vi "AutoBurn-BMU.vi"(0 "类型":u32(ring)=4 items=["PCI5121"=1, "PCI9810"=2, "USBCAN1"=3, "USBCAN2"=4, "PCI9820"=5, "CAN232"=6, "PCI5110"=7, "CANLite(mini)"=8, "ISA9620"=9, "ISA5420"=10, "PC104CAN"=11, "CANET"=17, "DNP9810"=13, "USBCAN-E-U"=20, "USBCAN-2E-U"=21], 1 "MyIndex":i32, 5 "波特率":T2(ring)=enum."500Kbps", 7 "设备索引":u32(ring) items=["0", "1", "2", "3", "4", "5", "6", "7", "8", "9", "10", "11", "12", "13", "14", "15", ""], 9 "CAN路数":u32(ring) items=["0", "1"], 11 "请选择板号":u16(ring)=1 items=["BMU1"=1, "BMU2"=2, "BMU3"=3, "BMU4"=4, "BMU5"=5, "BMU6"=6, "BMU7"=7, "BMU8"=8, "BMU9"=9, "BMU10"=10, "BMU11"=11, "BMU12"=12, "BMU13"=13, "BMU14"=14, "BMU15"=15, "BMU16"=16, "BMU17"=17, "BMU18"=18, "BMU19"=19, "BMU20"=20], 12 "板类型":enum16{"BCU/主板", "BMU/从板"}(ring)) -> ()   [LabVIEW 2013]
uses:
  <vilib>/Utility/config.llb/Write Key (String).vi
  <vilib>/Utility/config.llb/Read Key (String).vi
  <vilib>/Utility/file.llb/Read From Spreadsheet File (string).vi
  Settings/ControlCAN.dll
  <vilib>/Utility/config.llb/NI_LVConfig.lvlib
panel:
  out "退出？(T)":bool=TRUE
  out "VCI_CAN_OBJ_R 2":T1 {"ID" format="%x"}
  out "结果":bool
  in  "波特率 2":T2(ring)=enum."500Kbps"
  in  "错误输入（无错误）":errorcluster
  out "开始下载数据":u32
  out "开始下载数据":bool=TRUE
  out "耗时：":u32
  out "start":u32
  out "update flag":bool=TRUE
  in  "目标板类型":enum16{"BCU/主板", "BMU/从板"}(ring)
  out "Random":u32
  out "CRC16":u16 format="%x"
  out "进入烧录":bool
  out "boot模式应答计数":i32
  out "boot模式应答...成功":bool=TRUE
  out "总行数":i32
  in  "错误输入（无错误） 7":errorcluster caption="错误输入（无错误）"
  out "错误输出 18":errorcluster caption="错误输出"
  out "当前发送行":i32
  in  "错误输入（无错误） 6":errorcluster caption="错误输入（无错误）"
  out "错误输出 17":errorcluster caption="错误输出"
  in  "错误输入（无错误） 5":errorcluster caption="错误输入（无错误）"
  out "错误输出 16":errorcluster caption="错误输出"
  in  "错误输入（无错误） 4":errorcluster caption="错误输入（无错误）"
  out "错误输出 15":errorcluster caption="错误输出"
  in  "错误输入（无错误） 3":errorcluster caption="错误输入（无错误）"
  out "错误输出 14":errorcluster caption="错误输出"
  out "错误输出 13":errorcluster caption="错误输出"
  out "错误输出 12":errorcluster caption="错误输出"
  out "总电压":dbl
  out "Life":dbl
  out "Info：":string
  in  "手动进入编程模式 2":bool
  out "T9":bool=TRUE
  out "T8":u8
  out "T7":bool=TRUE
  out "T6":bool=TRUE
  out "T5":bool=TRUE
  out "T4":bool=TRUE
  out "T3":bool=TRUE
  out "T2":bool=TRUE
  out "T1":bool=TRUE
  out "错误输出 3":errorcluster caption="错误输出"
  in  "Monitor":bool
  out "校验":bool
  in  "手动进入编程模式":bool
  in  "板类型":enum16{"请选择板类型", "主板", "从板", "高压板"}(ring)=enum."主板"
  out "烧录结果":bool=TRUE
  out "擦除完成":bool
  out "进入烧录模式":bool
  out "MD5校验":bool
  out "进度":u8(slide) scale=0.0..100.0
  out "校验码实际值":string
  in  "校验码期望值":string
  in  "应用程序路径":path
  out "连接状态":bool=TRUE
  in  "滤波方式":u8(ring) items=["Dual Filter", "Single Filter"]
  in  "工作方式":u8(ring) items=["Normal", "Listen Only"]
  in  "开始监控":bool
  out "CAN数据":bool
  out "Monitor_flag":bool
  out "PC端-协议类型 2":enum16{"TCP服务器Server", "TCP客户端Client"}(ring)
  out "通信端口:":u32
  out "CANET地址格式如：192.168.0.178":string
  out "发送数据长度":dbl
  out "发送的数据":i32[](array[numeric])
  in  "设备索引 4":u16(ring) items=["0", "1", "2", "3", "4", "5", "6", "7", "8", "9", "10", "11", "12", "13", "14", "15", ""]
  in  "CAN路数 4":u16(ring) items=["0", "1"]
  in  "设备类型 4":u16(ring)=4 items=["PCI5121"=1, "PCI9810"=2, "USBCAN1"=3, "USBCAN2"=4, "PCI9820"=5, "CAN232"=6, "PCI5110"=7, "CANLite(mini)"=8, "ISA9620"=9, "ISA5420"=10, "PC104CAN"=11, "CANETE"=12, "DNP9810"=13]
  out "Mode":bool
  in  "开始监控 2":bool
  out "大小":i32=426
  out "地址长度 2":u32=4
  out "数据长度 2":u32=64
  out "子字符串 2":string="9B2F9B349B399B3E9B439B499B4F9B559B5B9B619B679B6D9B739B799B7F7C7B"
  out "数据长度":u32=64
  out "地址长度":u32=4
  in  "设定":bool
  out "VCI_CAN_OBJ_T":T1 {"ID" format="%x"}
  out "子数组":string[](array[string])
  in  "从板号":dbl
  out "从板号2":dbl
  in  "读取":bool
  out "TEMP":bool
  out "CAN状态 2":bool
  out "VCI_CAN_OBJ_R":T1={"ID"=0, "TimeStamp"=0, "TimeFlag"=0, "SendType"=1, "RemoteFlag"=0, "ExternFlag"=0, "DataLen"=8, 0, 0, 0, 0, 0, 0, 0, 0, 0, 0, 0}
  out "接收":T1={"ID"=0, "TimeStamp"=61537964, "TimeFlag"=1, "SendType"=250, "RemoteFlag"=0, "ExternFlag"=0, "DataLen"=1, 255, 0, 0, 0, 0, 0, 0, 0, 0, 0, 124} {"ID" min=2 max=104373490 step=1 format="%x"; "TimeStamp" min=1962977793 max=3175728; "TimeFlag" min=1 max=0; "SendType" max=131 step=11; "RemoteFlag" min=52 max=6 step=1; "ExternFlag" max=0; "DataLen" min=1 max=170; "?" min=117 max=48 step=117; "?" min=48 max=0; "?" max=0; "?" min=2 max=0; "?" max=150 step=11; "?" min=52 max=6 step=1; "?" max=0; "?" min=1 max=170; "?" min=120 max=175; "?" max=12; "?" max=0}
  out "收到请求":bool=TRUE
  out "分配":bool
  out "设置中？ 2":bool
  in  "Boar_Type":bool
  out "temp1":bool
  out "设置中？":bool
  in  "总步骤":dbl=21.0
  in  "失败重测次数":dbl=3.0
  out "一键测试":bool
  out "测试结果":bool
  in  "行号":dbl=21.0
  in  "工作方式 2":u8(ring) items=["Normal", "Listen Only"]
  in  "设备类型 2":u16(ring)=4 items=["PCI5121"=1, "PCI9810"=2, "USBCAN1"=3, "USBCAN2"=4, "PCI9820"=5, "CAN232"=6, "PCI5110"=7, "CANLite(mini)"=8, "ISA9620"=9, "ISA5420"=10, "PC104CAN"=11, "CANETE"=12, "DNP9810"=13]
  out "CAN状态":bool=TRUE
  in  "监控":bool
  # "当前BMU信息"
  # "蓝微新源BMS_CAN应用程序下载器V1.0.7D"
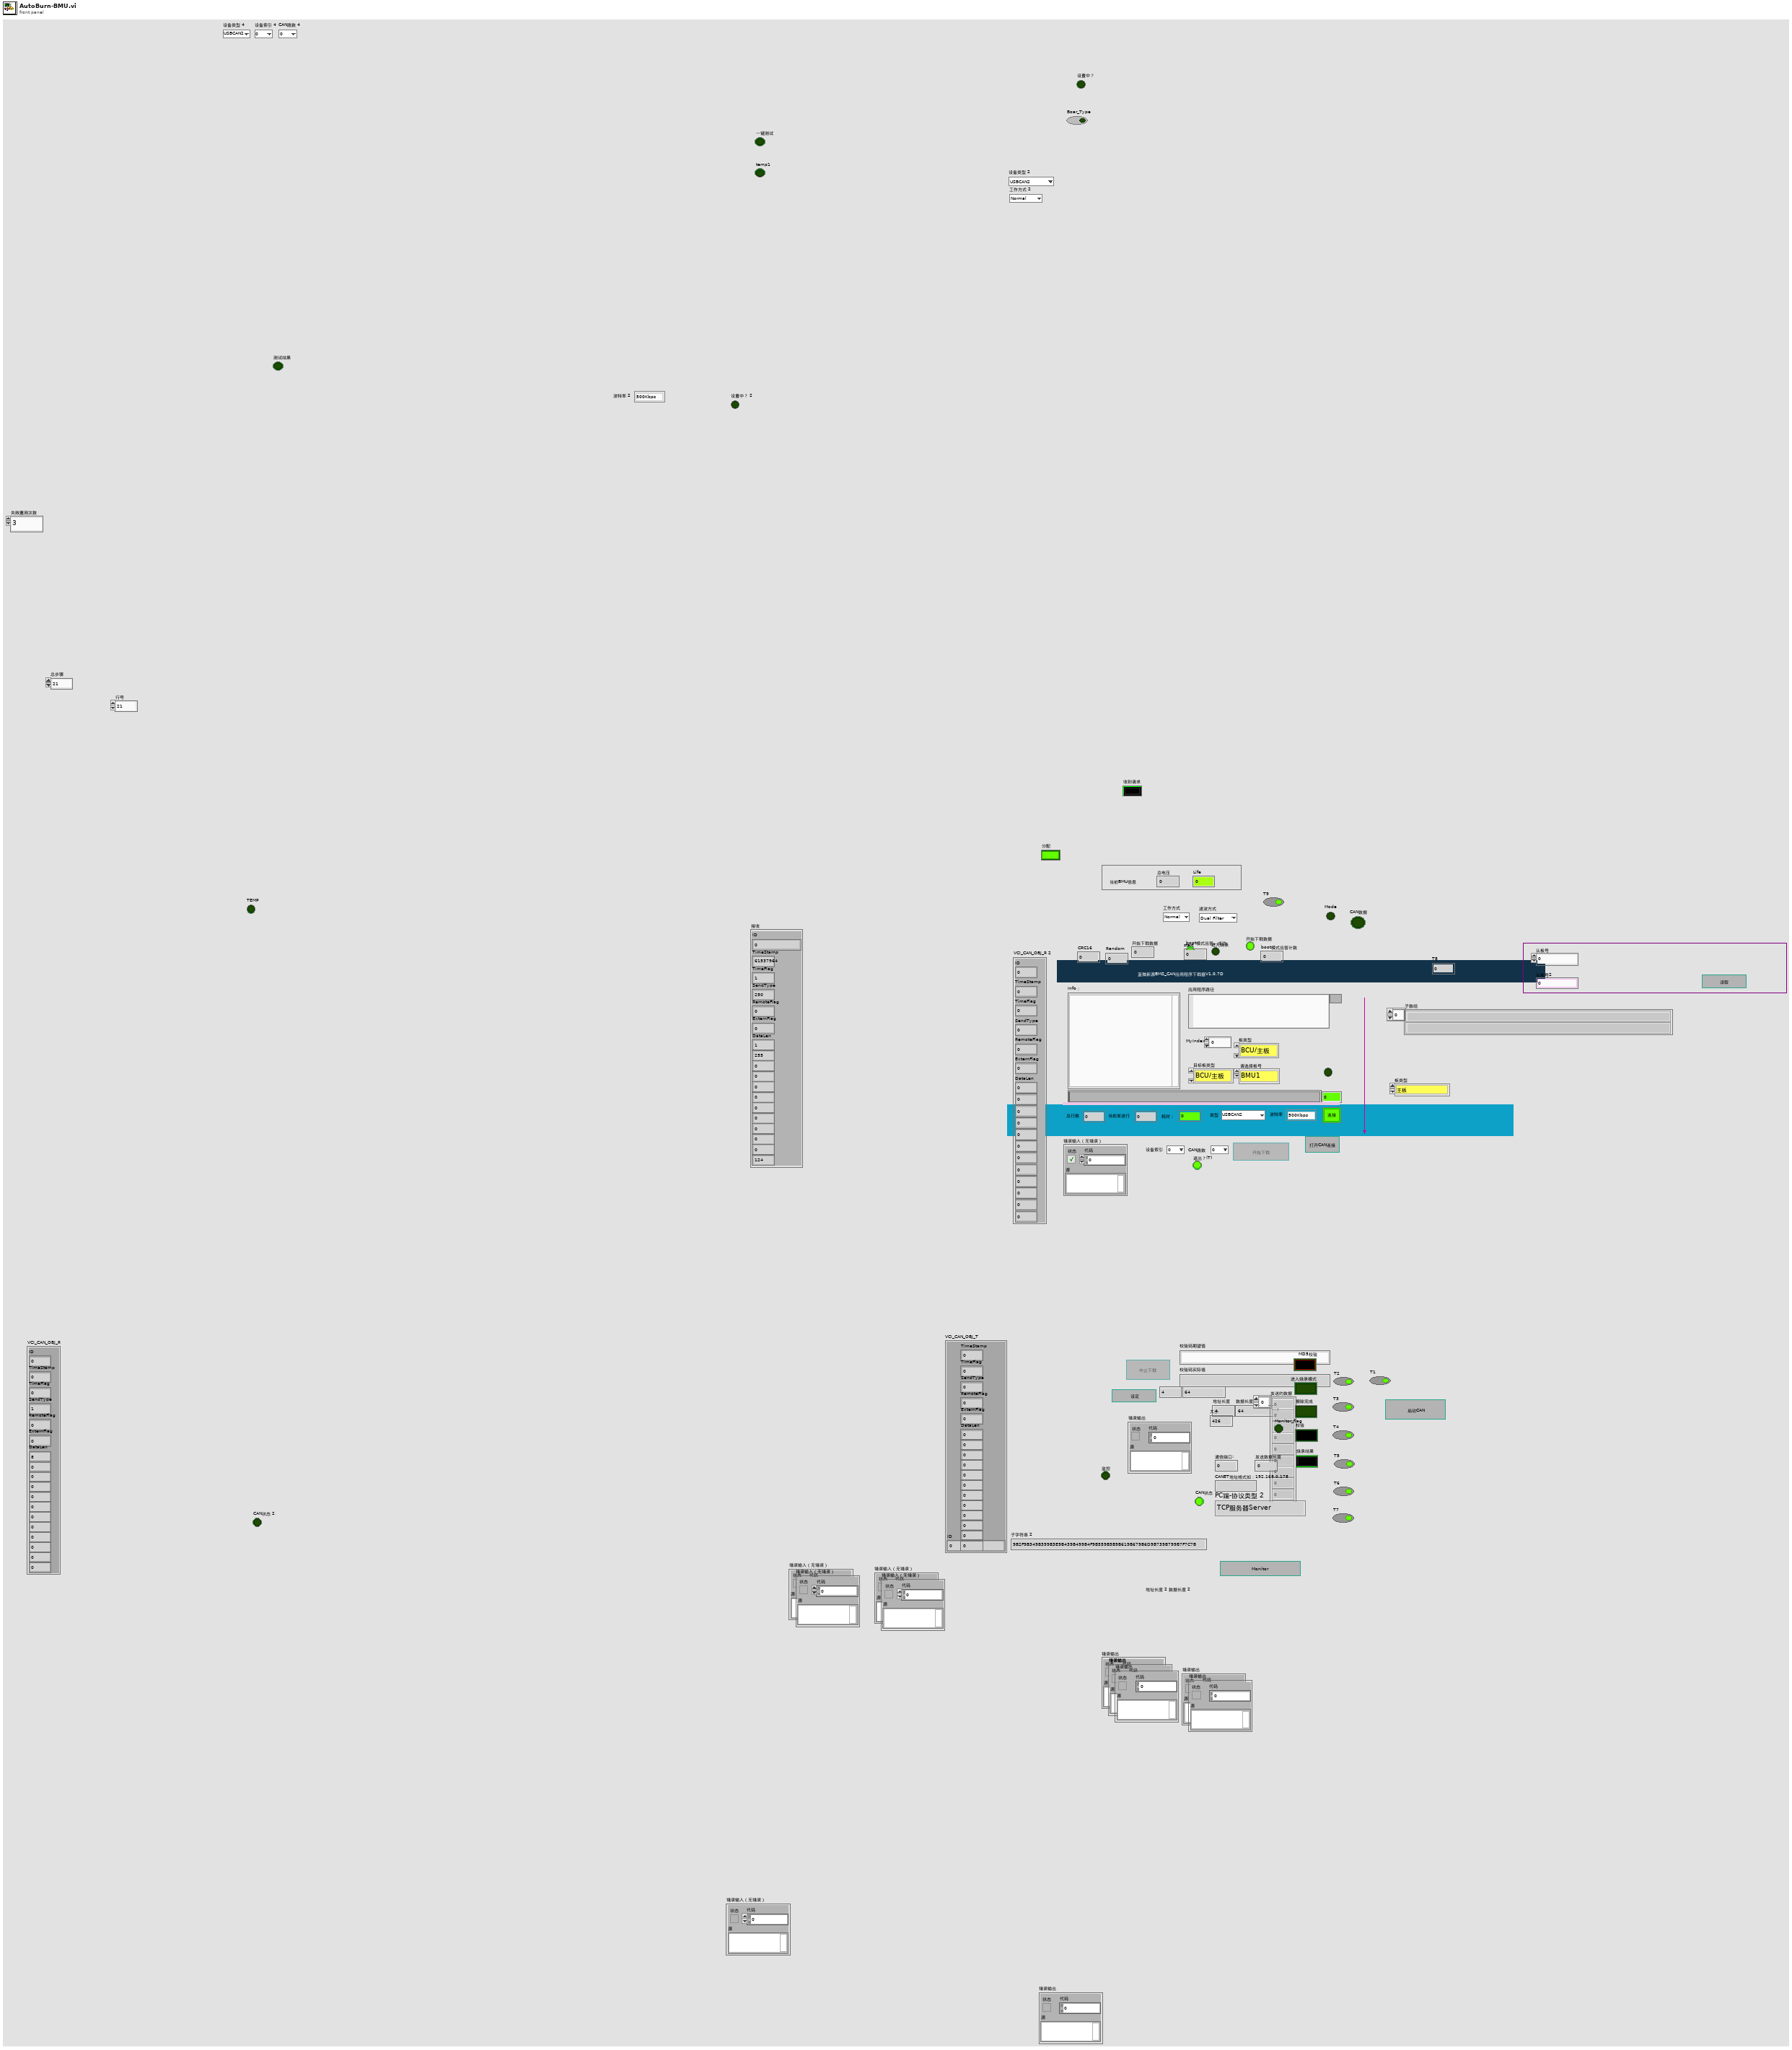
[diagram p1: front panel]
types:
  T1 = cluster{"ID":u32, "TimeStamp":u32, "TimeFlag":u8, "SendType":u8, "RemoteFlag":u8, "ExternFlag":u8, "DataLen":u8, u8, u8, u8, u8, u8, u8, u8, u8, u8, u8, u8}
  T2 = enum16{"5Kbps", "10Kbps", "20Kbps", "40Kbps", "50Kbps", "80Kbps", "100Kbps", "125Kbps", "200Kbps", "250Kbps", "400Kbps", "500Kbps", "666Kbps", "800Kbps", "1000Kbps"}
  T3 = enum8{"Enabled", "Disabled", "Disabled and Grayed Out"}
  T4 = typedef "NI_LVConfig.lvlib/Config Data RefNum.ctl" = refnum<k1>
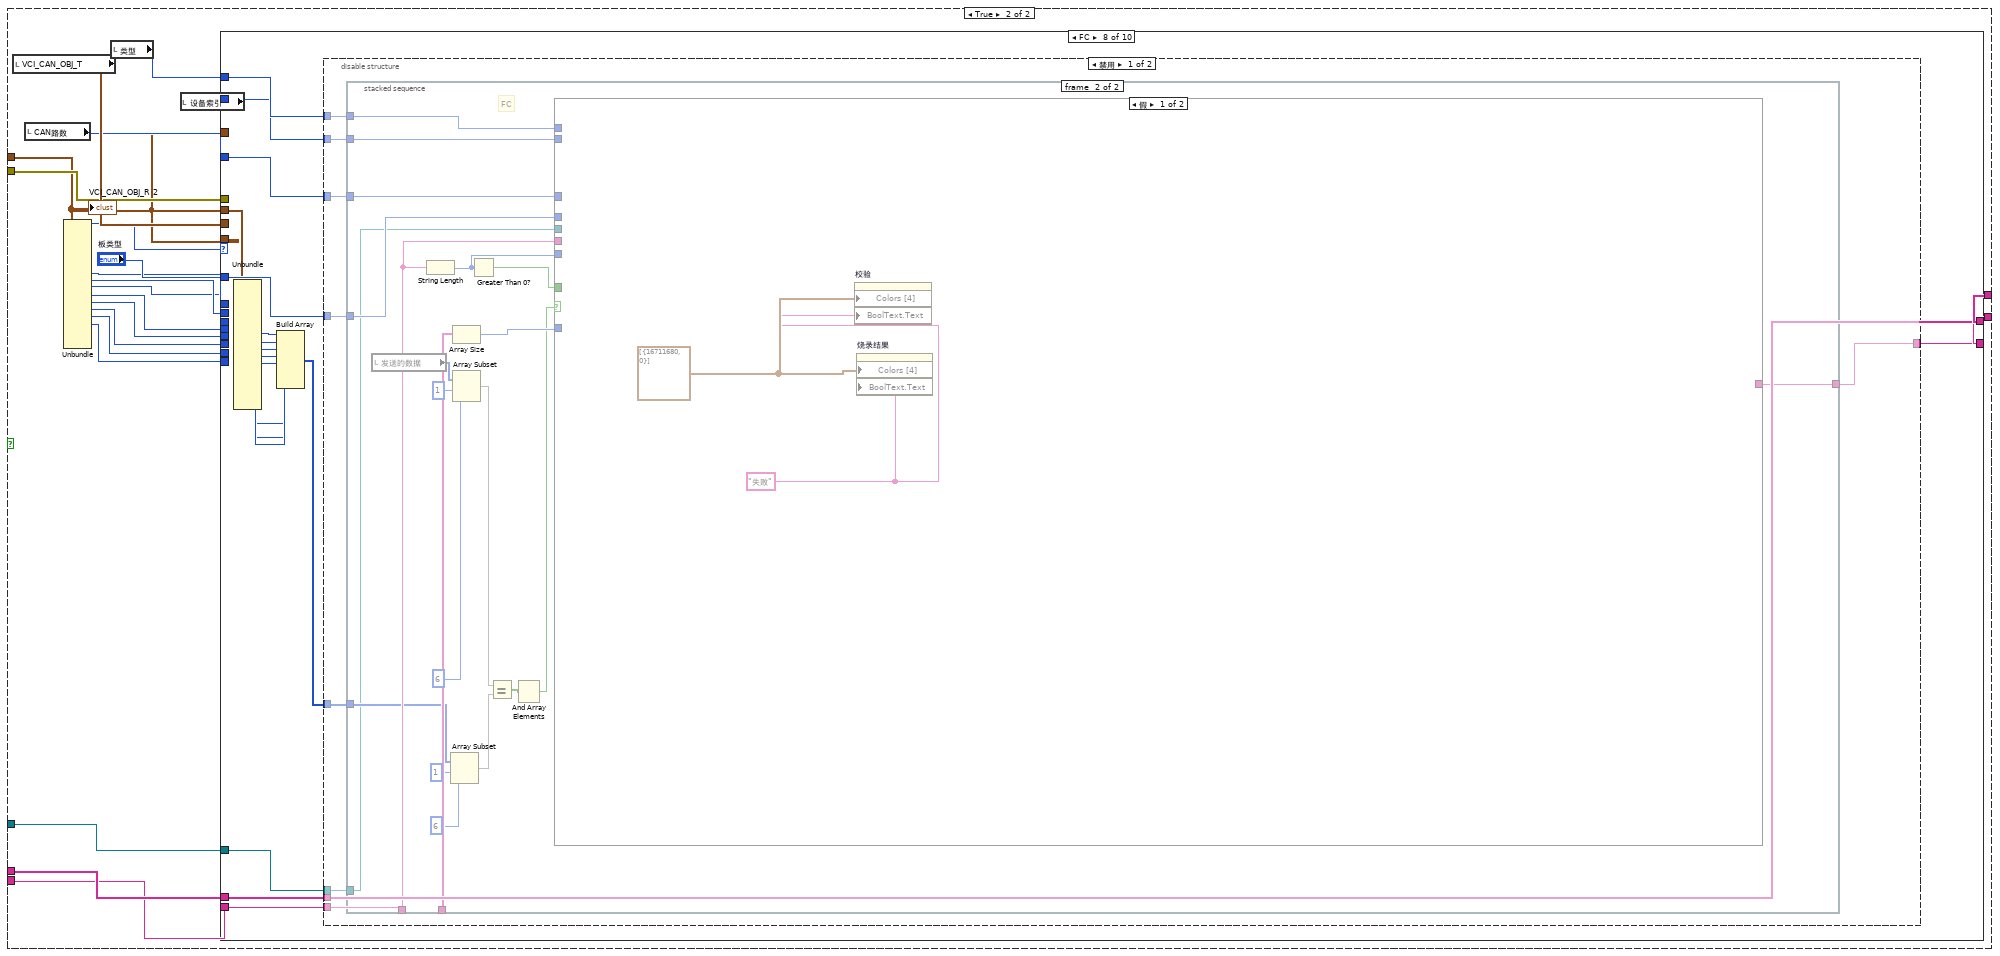
[diagram p2: hidden frame]
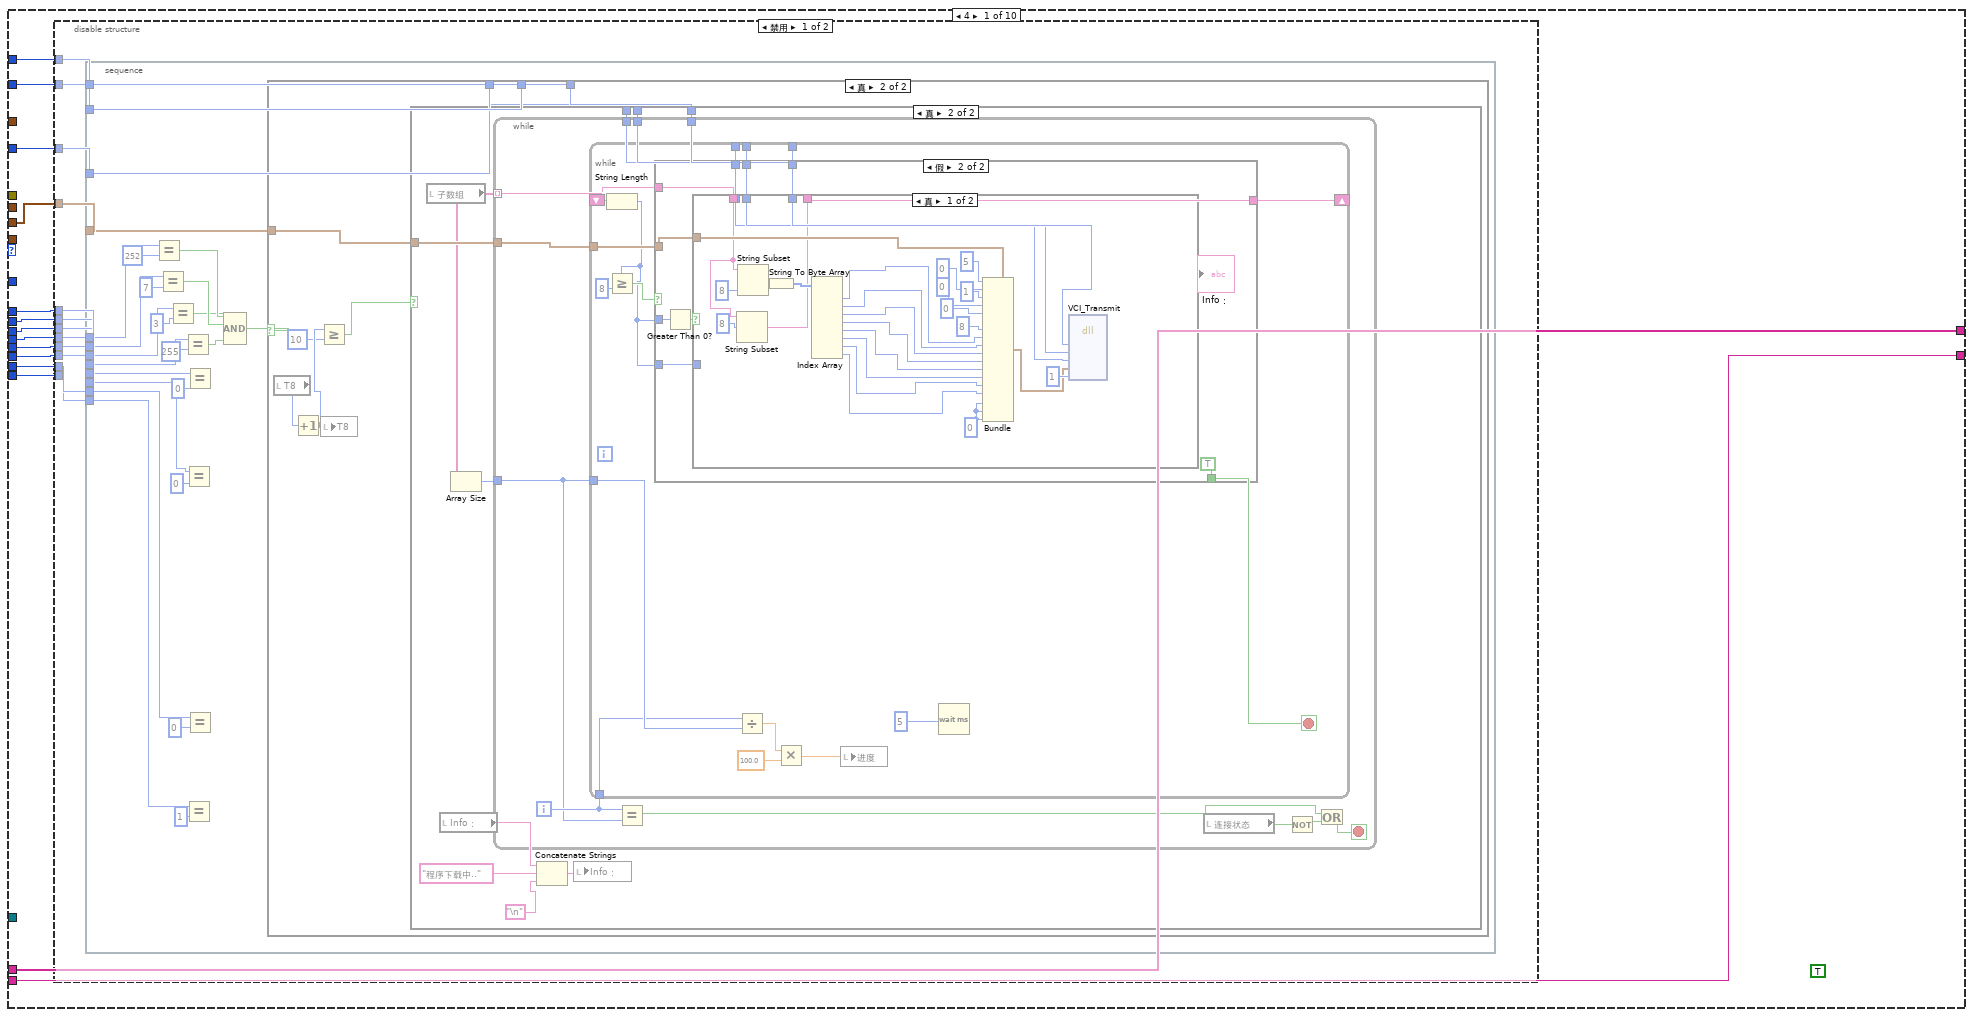
[diagram p3: hidden frame]
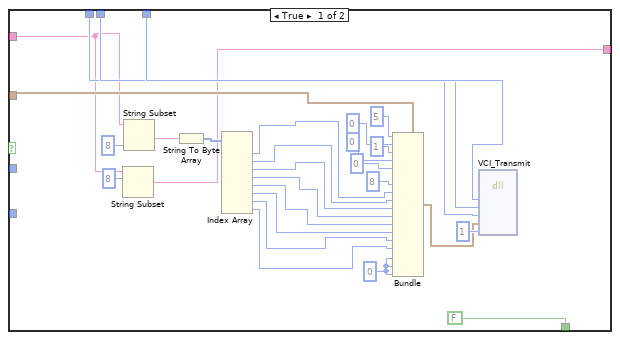
[diagram p6: hidden frame]
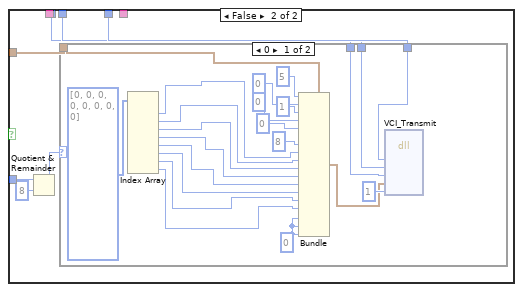
[diagram p7: hidden frame]
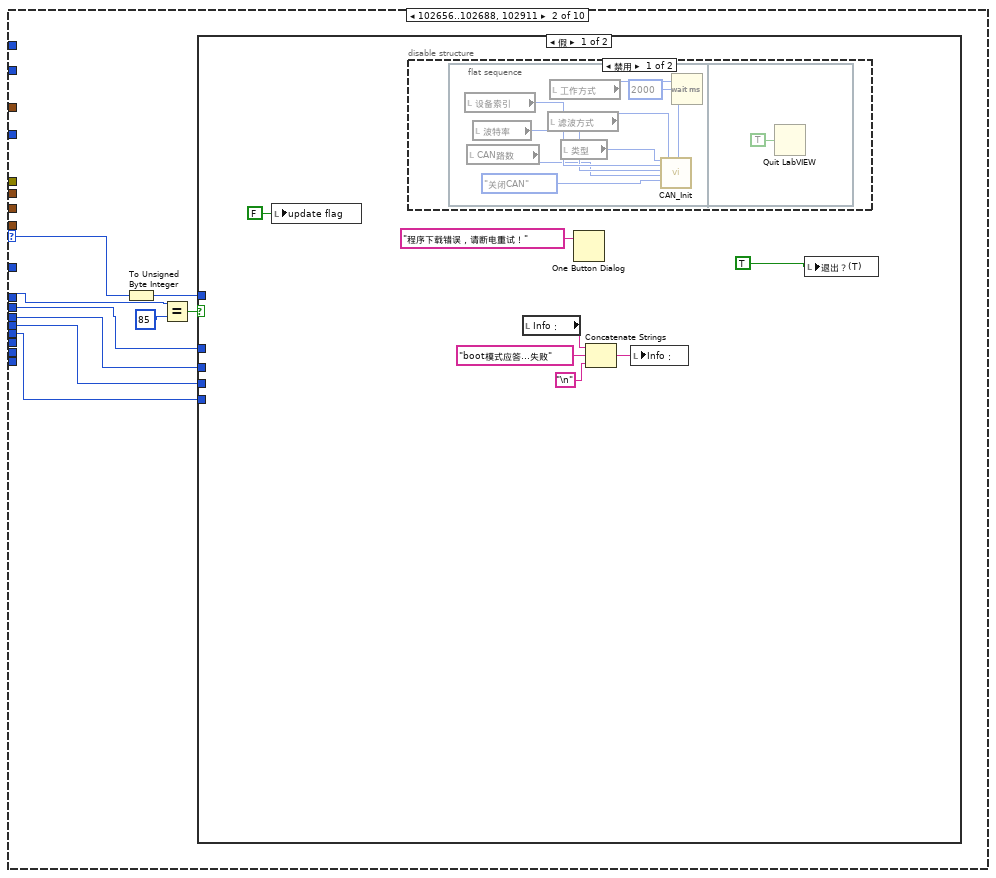
[diagram p10: hidden frame]
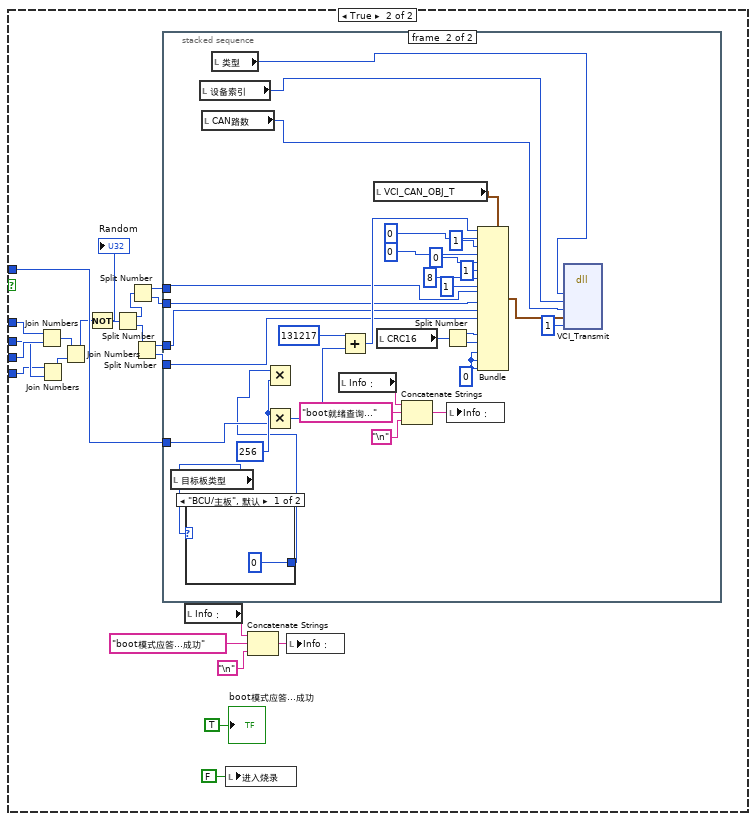
[diagram p12: hidden frame]
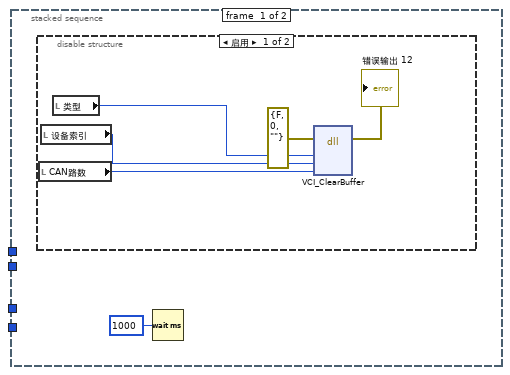
[diagram p13: hidden frame]
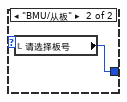
[diagram p15: hidden frame]
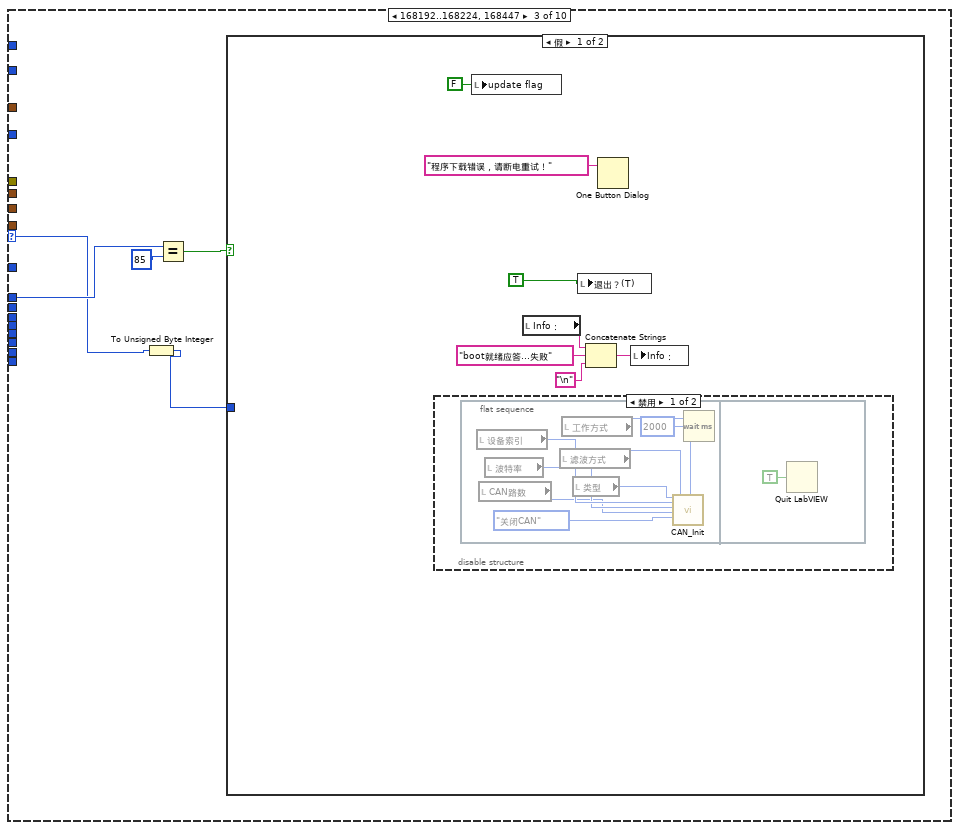
[diagram p16: hidden frame]
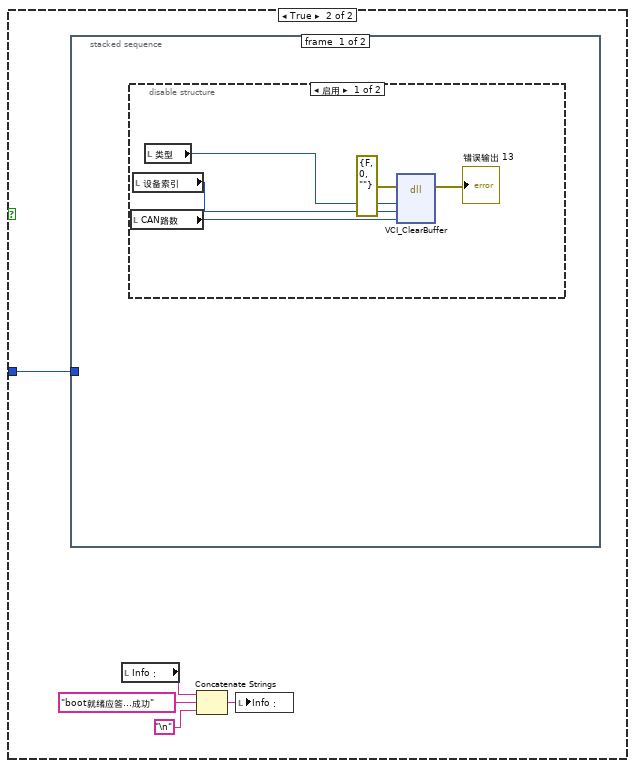
[diagram p18: hidden frame]
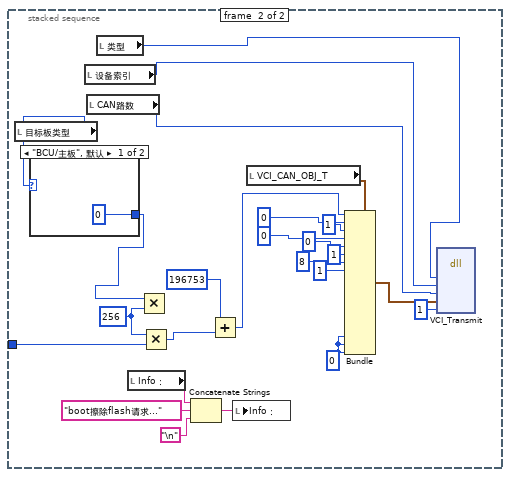
[diagram p20: hidden frame]
diagram:
  w7 = FALSE ("CAN状态")
  (unwired) u32 0
  (unwired) u32 255
  w26 = "" ("布尔文本.文本")
  w27 = cluster{u32, u32}[] [{0, 0}] ("颜色[4]")
  w34 = "" ("校验码期望值")
  w42 = FALSE ("进入烧录模式")
  n1 = local write "TEMP"(FALSE ("TEMP")) -> ()
  n2 = local write "校验码期望值"(w34) -> ()
  n3 = local write "校验码实际值"(w34) -> ()
  n4 = property on="校验" class="Bool (严格)"("Colors [4]"=w27, "BoolText.Text"=w26) -> ()  [unwired: 2 in, 2 out]
  n5 = property on="烧录结果" class="Bool (严格)"("Colors [4]"=w27, "BoolText.Text"=w26) -> ()  [unwired: 2 in, 2 out]
  n6 = local write "连接状态"(FALSE ("连接状态")) -> ()
  n7 = Number To Decimal String(number="MyIndex") -> (decimal integer string=w2:string)  [unwired: 1 in]
  n8 = local read "VCI_CAN_OBJ_R"() -> (w24:T1)
  n9 = Concatenate Strings("CAN" ("名称（未命名）"), w2) -> (w1:string)
  n10 = local write "boot模式应答...成功"(FALSE ("boot模式应答...成功")) -> ()
  n11 = local write "开始下载数据"(u32 0 ("开始下载数据")) -> ()
  n12 = local write "耗时："(u32 0 ("耗时：")) -> ()
  n13 = property on="请选择板号" class="Ring (严格)"("Visible"=TRUE ("可见")) -> ()  [unwired: 2 in, 2 out]
  n14 = local write "耗时："(u32 0 ("耗时：")) -> ()
  n15 = Initialize Array("", 1 ("维数大小")) -> (w38:string[])
  n16 = Obtain Queue(name (unnamed)=w1, element data type=w24, error in (no error)="错误输入（无错误）") -> (queue out=w25:refnum<queue>, error out=w12:errorcluster)  [unwired: 2 in, 1 out]
  n17 = while {
    tunnel: "错误输入（无错误）" -> [w45]
    tunnel: w25 -> [w47]
    stop <- w44 stop-if-true
    n18 = event shown="[0] 超时" {
      selector: _ -> [_ _ _ _ _ _ _ _ _ _ _]
      dyn-events: _ -> [_ _ _ _ _ _ _ _ _ _ _]
      timeout: 200 -> [_ _ _ _ _ _ _ _ _ _ _]
      tunnel: w45 -> [_ w146 _ _ w208 _ _ _ _ _ _]
      tunnel: w47 -> [_ _ _ _ _ _ _ _ w321 _ _]
      event Timeout {
        n19 = event-data() -> ()  [unwired: 1 in, 2 out]
        n20 = local read "开始下载数据"() -> (w54:bool)
        n21 = local read "update flag"() -> (w55:bool)
        n22 = case shown="真" w55 {
          frame False {
          }
          frame True {
            n23 = local read "start"() -> (w80:u32)
            n24 = Tick Count (ms)() -> (millisecond timer value=w81:u32)
            n25 = Subtract(x=w81, y=w80) -> (x-y=w79:u32)
            n26 = local read "目标板类型"() -> (w77:enum16{"BCU/主板", "BMU/从板"})
            n27 = Divide(x=w79, y=u32 1000) -> (x/y=w76:dbl)
            "耗时：" <- w76
            n28 = To Unsigned Long Integer(number=w76) -> (unsigned 32bit integer=w75:u32)
            n29 = case shown="\"BMU/从板\"" w77 {
              tunnel: w75 -> [w84 w101]
              frame "BCU/主板", Default {
                n30 = Equal?(x=w84, y=80.0) -> (x = y?=w82:bool)
                n31 = case shown="真" w82 {
                  frame False {
                  }
                  frame True {
                    n32 = local read "Info："() -> (w87:string)
                    n33 = local write "update flag"(FALSE ("update flag")) -> ()
                    n34 = local write "退出？(T)"(TRUE ("退出？(T)")) -> ()
                    n35 = Concatenate Strings(w87, "超时请重试" ("字符串")) -> (w88:string)
                    n36 = local write "Info："(w88) -> ()
                    n37 = disable-structure shown="禁用" {
                      frame Disabled {
                        n38 = flat-sequence {
                          frame #0 {
                            n39 = local read "设备索引"() -> (w96:u32)
                            n40 = local read "CAN路数"() -> (w94:u32)
                            n41 = local read "波特率"() -> (w95:T2)
                            n42 = local read "滤波方式"() -> (w93:u8)
                            n43 = local read "工作方式"() -> (w92:u8)
                            n44 = local read "类型"() -> (w97:u32)
                            n45 = call "CAN_Init.vi"("设备类型"=w97, "设备索引"=w96, "波特率"=w95, "CAN路数"=w94, "操作类型"=enum16{"初始化CAN", "关闭CAN"}."关闭CAN", 6:w93, 10:w92) -> ()  [unwired: 12 in, 1 out]
                            n46 = Wait (ms)(milliseconds to wait=u32 2000 ("等待时间（毫秒）")) -> ()  [unwired: 1 out]
                          }
                          frame #1 {
                            n47 = Quit LabVIEW(quit? (T)=TRUE ("退出？(T)")) -> ()
                          }
                        }
                      }
                      frame Enabled {
                      }
                    }
                  }
                }
              }
              frame "BMU/从板" {
                n48 = Equal?(x=w101, y=50.0) -> (x = y?=w99:bool)
                n49 = case shown="真" w99 {
                  frame False {
                  }
                  frame True {
                    n50 = local read "Info："() -> (w103:string)
                    n51 = local write "update flag"(FALSE ("update flag")) -> ()
                    n52 = Concatenate Strings(w103, "超时请重试\n" ("字符串")) -> (w104:string)
                    n53 = local write "Info："(w104) -> ()
                    n54 = flat-sequence {
                      frame #0 {
                        n55 = local write "退出？(T)"(TRUE ("退出？(T)")) -> ()
                        n56 = Wait (ms)(milliseconds to wait=u32 2000 ("等待时间（毫秒）")) -> ()  [unwired: 1 out]
                      }
                      frame #1 {
                      }
                    }
                  }
                }
              }
            }
          }
        }
        n57 = case shown="真" w54 {
          frame False {
          }
          frame True {
            n58 = local read "开始下载数据"() -> (w67:u32)
            n59 = Tick Count (ms)() -> (millisecond timer value=w68:u32)
            n60 = Subtract(x=w68, y=w67) -> (x-y=w66:u32)
            n61 = Divide(x=w66, y=u32 1000) -> (x/y=w62:dbl)
            n62 = To Unsigned Long Integer(number=w62) -> (unsigned 32bit integer=w61:u32)
            n63 = Equal?(x=w61, y=3.0) -> (x = y?=w63:bool)
            n64 = case shown="真" w63 {
              frame False {
              }
              frame True {
                n65 = flat-sequence {
                  frame #0 {
                    n66 = local read "Info："() -> (w71:string)
                    n67 = local write "update flag"(FALSE ("update flag")) -> ()
                    n68 = Concatenate Strings(w71, "数据传输中断！\n" ("字符串")) -> (w70:string)
                    n69 = local write "Info："(w70) -> ()
                  }
                  frame #1 {
                  }
                  frame #2 {
                    n70 = local write "退出？(T)"(TRUE ("退出？(T)")) -> ()
                  }
                  frame #3 {
                    n71 = disable-structure shown="禁用" {
                      frame Disabled {
                        n72 = Quit LabVIEW(quit? (T)=TRUE ("退出？(T)")) -> ()
                      }
                      frame Enabled {
                      }
                    }
                  }
                }
              }
            }
          }
        }
        n73 = local read "boot模式应答...成功"() -> (w58:bool)
        n74 = local read "进入烧录"() -> (w56:bool)
        n75 = local read "boot模式应答计数"() -> (w60:i32)
        n76 = Increment(x=w60) -> (x+1=w48:i32)
        n77 = Equal?(x=25.0, y=w48) -> (x = y?=w52:bool)
        n78 = Equal?(x=w48, y=7) -> (x = y?=w50:bool)
        n79 = Not(x=w58) -> (.not. x?=w57:bool)
        n80 = Compound Arithmetic op=OR(w50, w52) -> (w49:bool)
        n81 = local write "boot模式应答计数"(w48) -> ()
        n82 = Compound Arithmetic op=AND(w49, w57, w56) -> (w59:bool)
        "结果" <- w59
        n83 = case shown="真" w59 {
          frame False {
          }
          frame True {
            n84 = local read "目标板类型"() -> (w109:enum16{"BCU/主板", "BMU/从板"})
            n85 = case shown="\"BMU/从板\"" w109 {
              tunnel: [u16 0 ("请选择板号") w121] -> w108
              frame "BCU/主板", Default {
              }
              frame "BMU/从板" {
                n86 = local read "请选择板号"() -> (w121:u16)
              }
            }
            n87 = Multiply(x=w108, y=u16 256) -> (x*y=w112:u16)
            n88 = Add(x=u32 65681 ("ID"), y=w112) -> (x+y=w110:u32)
            n89 = local read "VCI_CAN_OBJ_T"() -> (w114:T1)
            n90 = case shown="1, 默认" w108 {
              tunnel: [w126 w138] -> w118
              tunnel: w114 -> [w125 w137]
              tunnel: w110 -> [w123 w135]
              frame 0 {
                w122 = u8 170
                w129 = u8 0 ("元素")
                n91 = Bundle(cluster=w125, "ID"=w123, "TimeStamp"=u8 0 ("RemoteFlag"), "TimeFlag"=u8 1, "SendType"=u8 0 ("DataLen"), "RemoteFlag"=u8 0, "ExternFlag"=u8 1, "DataLen"=u8 8, u8 1 ("元素"), w122, w122, w122, w122, w129, w129, w129) -> (w126:T1)  [unwired: 3 in]
              }
              frame 1, Default {
                w134 = u8 187
                w141 = u8 0 ("元素")
                n92 = Bundle(cluster=w137, "ID"=w135, "TimeStamp"=u8 0 ("RemoteFlag"), "TimeFlag"=u8 1, "SendType"=u8 0 ("DataLen"), "RemoteFlag"=u8 0, "ExternFlag"=u8 1, "DataLen"=u8 8, u8 1 ("元素"), w134, w134, w134, w134, w141, w141, w141) -> (w138:T1)  [unwired: 3 in]
              }
            }
            n93 = local read "设备索引"() -> (w116:u32)
            n94 = local read "CAN路数"() -> (w115:u32)
            n95 = local read "类型"() -> (w117:u32)
            n96 = dll-call lib="F:/Bluewave New Energy/SVN_Work/AutoTest_TestStand/trunk/AutoTest_TestStand/Driver/ZlgCan/BHN01/AutoBurn/Settings/ControlCAN.dll" fn="VCI_Transmit"("DeviceType"=w117, "DeviceInd"=w116, "CANInd"=w115, "pSend"=w118, "Len"=u32 1) -> ()  [unwired: 5 in, 6 out]
          }
        }
      }
      event "开始监控": Value Change {
        n97 = event-data() -> ("NewVal"=w147:bool)  [unwired: 1 in, 5 out]
        n98 = disable-structure shown="禁用" {
          disable-tunnel: w147 -> [w152 _]
          disable-tunnel: w146 -> [w148 _]
          frame Disabled {
            n99 = local write "TEMP"(w152) -> ()
            n100 = local read "通信端口:"() -> (w149:u32)
            n101 = local read "CANET地址格式如：192.168.0.178"() -> (w151:string)
            n102 = local read "设备索引"() -> (w154:u32)
            n103 = local read "CAN路数"() -> (w156:u32)
            n104 = local read "波特率"() -> (w155:T2)
            n105 = local read "滤波方式"() -> (w157:u8)
            n106 = local read "工作方式"() -> (w158:u8)
            n107 = local read "类型"() -> (w153:u32)
            n108 = local read "PC端-协议类型 2"() -> (w150:enum16{"TCP服务器Server", "TCP客户端Client"})
            n109 = case shown="真" w152 {
              tunnel: w153 -> [w177 w201]
              tunnel: w154 -> [w176 w200]
              tunnel: w155 -> [w175 w199]
              tunnel: w156 -> [w174 w198]
              tunnel: w157 -> [w172 w196]
              tunnel: w158 -> [w171 w195]
              tunnel: w151 -> [w165 w193]
              tunnel: w150 -> [w164 w192]
              tunnel: w149 -> [w163 w191]
              tunnel: w148 -> [w162 _]
              frame True {
                w159 = T3."Enabled" ("禁用")
                w167 = "" ("布尔文本.文本")
                w168 = cluster{u32, u32}[] [{0, 0}] ("颜色[4]")
                w169 = FALSE
                n110 = call "CAN_Init.vi"("设备类型"=w177, "设备索引"=w176, "波特率"=w175, "CAN路数"=w174, "操作类型"=enum16{"初始化CAN", "关闭CAN"}."初始化CAN", 5:w162, 6:w172, 8:w165, 9:w163, 10:w171, 12:w164) -> ("CAN 操作结果"=w160:bool, 19:w161)  [unwired: 7 in]
                n111 = local write "Monitor_flag"(FALSE ("Monitor_flag")) -> ()
                n112 = invoke on="Monitor" class="Bool" method="Reinit To Default"(error in=w161) -> ()  [unwired: 2 in, 3 out]
                n113 = local write "进度"(u8 0 ("进度")) -> ()
                n114 = local write "CAN状态"(w160) -> ()
                n115 = local write "连接状态"(w160) -> ()
                n116 = local write "擦除完成"(w169) -> ()
                n117 = local write "进入烧录模式"(w169) -> ()
                n118 = property on="烧录结果" class="Bool (严格)"("Colors [4]"=w168, "BoolText.Text"=w167) -> ()  [unwired: 2 in, 2 out]
                n119 = property on="校验" class="Bool (严格)"("Colors [4]"=w168, "BoolText.Text"=w167) -> ()  [unwired: 2 in, 2 out]
                n120 = local write "烧录结果"(w169) -> ()
                n121 = case shown="真" w160 {
                  frame True {
                    n122 = local read "Info："() -> (w178:string)
                    n123 = Concatenate Strings(w178, "启动CAN成功.." ("字符串"), "\n") -> (w181:string)
                    n124 = local write "Info："(w181) -> ()
                  }
                  frame False {
                    n125 = local read "Info："() -> (w182:string)
                    n126 = Concatenate Strings(w182, "启动CAN失败.." ("字符串"), "\n") -> (w185:string)
                    n127 = local write "Info："(w185) -> ()
                  }
                }
                n128 = property on="手动进入编程模式" class="Bool (严格)"("DisabledEnum"=w159) -> ()  [unwired: 2 in, 2 out]
                n129 = property on="中止编程模式 2" class="Bool (严格)"("DisabledEnum"=w159) -> ()  [unwired: 2 in, 2 out]
              }
              frame False {
                w186 = T3."Disabled and Grayed Out" ("禁用")
                w194 = FALSE ("CAN状态")
                n130 = call "CAN_Init.vi"("设备类型"=w201, "设备索引"=w200, "波特率"=w199, "CAN路数"=w198, "操作类型"=enum16{"初始化CAN", "关闭CAN"}."关闭CAN", 6:w196, 8:w193, 9:w191, 10:w195, 12:w192) -> ()  [unwired: 9 in, 1 out]
                n131 = local write "CAN状态"(w194) -> ()
                n132 = local write "连接状态"(w194) -> ()
                n133 = property on="手动进入编程模式" class="Bool (严格)"("DisabledEnum"=w186) -> ()  [unwired: 2 in, 2 out]
                n134 = property on="中止编程模式" class="Bool (严格)"("DisabledEnum"=w186) -> ()  [unwired: 2 in, 2 out]
                n135 = Concatenate Strings("" ("字符串"), "关闭CAN成功..." ("字符串"), "\n") -> (w190:string)
                n136 = local write "Info："(w190) -> ()
              }
            }
          }
          frame Enabled {
          }
        }
      }
      event "Info：": Shortcut Menu Selection (User) {
        n137 = event-data() -> ("ItemPath"=w202:string)  [unwired: 1 in, 7 out]
        n138 = case shown="\"清空\"" w202 {
          frame "假", Default {
          }
          frame "清空" {
            n139 = local write "Info："("" ("Info：")) -> ()
          }
        }
      }
      event Menu Selection (User) {
        n140 = event-data() -> ("ItemTag"=w205:string)  [unwired: 1 in, 6 out]
        n141 = case shown="\"烧录多块\"" w205 {
          tunnel: [FALSE ("Mode") TRUE ("Mode")] -> w204
          frame "烧录多块" {
          }
          frame "烧录一块", Default {
          }
        }
        n142 = local write "Mode"(w204) -> ()
      }
      event "类型": Value Change {
        n143 = event-data() -> ("NewVal"=w209:u32)  [unwired: 1 in, 5 out]
        n144 = case shown="17" w209 {
          tunnel: w208 -> [_ w213]
          frame 0, Default {
          }
          frame 17 {
            n145 = call "PortSet.vi"("error in (no error)"=w213) -> ("PC端-协议类型 2"=→"PC端-协议类型 2":enum16{"TCP服务器Server", "TCP客户端Client"}, "通信端口:"=→"通信端口:":dbl, "CANET地址格式如：192.168.0.178"=→"CANET地址格式如：192.168.0.178":string)  [unwired: 7 in, 1 out]
          }
        }
      }
      event "类型": Mouse Down {
        w214 = u16 4 items=["PCI5121"=1, "PCI9810"=2, "USBCAN1"=3, "USBCAN2"=4, "PCI9820"=5, "CAN232"=6, "PCI5110"=7, "CANLite(mini)"=8, "ISA9620"=9, "ISA5420"=10, "PC104CAN"=11, "CANET"=17, "DNP9810"=13] ("设备类型")
        n146 = event-data() -> ()  [unwired: 1 in, 8 out]
        n147 = local write "类型"(w214) -> ()
      }
      event "Monitor": Value Change {
        n148 = event-data() -> ("NewVal"=w218:bool)  [unwired: 1 in, 5 out]
        n149 = local read "板类型"() -> (w217:enum16{"请选择板类型", "主板", "从板", "高压板"})
        n150 = Equal?(x=w217, y=enum16{"请选择板类型", "主板", "从板", "高压板"}."请选择板类型") -> (x = y?=w215:bool)
        n151 = case shown="真" w215 {
          tunnel: w218 -> [w221 _]
          frame False {
            n152 = Select(t=0.0, s=w221, f=2.0) -> (s? t:f=w222:dbl)
            n153 = property on="手动进入编程模式" class="Bool (严格)"("Disabled"=w222) -> ()  [unwired: 2 in, 2 out]
            "Monitor_flag" <- w221
          }
          frame True {
            n154 = invoke on="Monitor" class="Bool" method="Reinit To Default"() -> ()  [unwired: 3 in, 3 out]
            n155 = One Button Dialog(message=" 请选择板的类型！！" ("消息")) -> ()  [unwired: 1 in, 1 out]
          }
        }
      }
      event "应用程序路径": Value Change {
        n156 = event-data() -> ("NewVal"=w225:path)  [unwired: 1 in, 5 out]
        n157 = Not A Number/Path/Refnum?(number/path/refnum=w225) -> (NaN/Path/Refnum?=w228:bool)
        n158 = Strip Path(path=w225) -> (name=w224:string)  [unwired: 1 out]
        n159 = String Subset(string=w224, offset (0)=6 ("偏移量(0)"), length (rest)=2 ("长度（剩余）")) -> (substring=w229:string)
        n160 = case shown="\"SS\"" w229 {
          tunnel: [TRUE ("y") FALSE ("y") FALSE ("y")] -> w226
          frame "假", Default {
            n161 = local read "Info："() -> (w233:string)
            n162 = Concatenate Strings(w233, "无法识别板类型！\n" ("字符串")) -> (w235:string)
            n163 = local write "Info："(w235) -> ()
          }
          frame "MS" {
            n164 = local read "Info："() -> (w237:string)
            n165 = local write "目标板类型"(enum16{"BCU/主板", "BMU/从板"}."BCU/主板" ("类型")) -> ()
            n166 = property on="请选择板号" class="Ring (严格)"("Visible"=FALSE ("可见")) -> ()  [unwired: 2 in, 2 out]
            n167 = Concatenate Strings(w237, "通过文件识别为主板！\n" ("字符串")) -> (w238:string)
            n168 = local write "Info："(w238) -> ()
          }
          frame "SS" {
            n169 = local read "Info："() -> (w243:string)
            n170 = local write "目标板类型"(enum16{"BCU/主板", "BMU/从板"}."BMU/从板" ("类型")) -> ()
            n171 = property on="请选择板号" class="Ring (严格)"("Visible"=TRUE ("可见")) -> ()  [unwired: 2 in, 2 out]
            n172 = Concatenate Strings(w243, "通过文件识别为从板！\n" ("字符串")) -> (w244:string)
            n173 = local write "Info："(w244) -> ()
          }
        }
        n174 = Or(x=w228, y=w226) -> (x .or. y?=w227:bool)
        n175 = case shown="假" w227 {
          tunnel: w225 -> [w283 _]
          frame False {
            n176 = Path To String(path=w283) -> (string=w257:string)
            n177 = local read "Info："() -> (w253:string)
            n178 = String Subset(string=w257, offset (0)=6 ("偏移量(0)"), length (rest)=2 ("长度（剩余）")) -> (substring=w254:string)
            n179 = call-poly <vilib>:"Read From Spreadsheet File.vi"("file path (dialog if empty)"=w283) -> ("all rows"=w285:string[][])  [unwired: 6 in, 4 out]
            n180 = call <vilib>:"Space Constant.vi"() -> ("String"=w281:string)
            n181 = Search and Replace String(replace all?=TRUE ("替换全部？(F)"), input string=w257, search string=w281, replace string="" ("替换字符串(\"\")")) -> (result string=w268:string)  [unwired: 4 in, 3 out]
            n182 = case shown="\"真\"" w254 {
              frame "假", Default {
              }
              frame "真" {
              }
            }
            n183 = Concatenate Strings(w253, "文件加载成功！\n" ("字符串")) -> (w251:string)
            n184 = Index Array(array=w285, index (col)=0 ("禁用的索引 (列)")) -> (element=w272:string[])  [unwired: 1 in]
            n185 = Search/Split String(string=w268, search string/char (-)="(MD5=" ("搜索字符串/字符(-)")) -> (match + rest of string=w265:string, offset of match=w275:i32)  [unwired: 1 in, 1 out]
            n186 = local write "Info："(w251) -> ()
            n187 = Delete From Array(array=w272, length=1 ("长度"), index=0 ("索引")) -> (array with subset deleted=w264:string[])  [unwired: 1 out]
            n188 = call <vilib>:"MD5Checksum File.vi"("Path"=w283) -> ("MD5 message-digest"=w248:string)  [unwired: 9 in, 1 out]
            n189 = Array Size(array=w264) -> (size(s)=w262:i32)
            n190 = Decrement(x=w262) -> (x-1=w261:i32)
            n191 = Delete From Array(array=w264, length=1 ("长度"), index=w261) -> (array with subset deleted=w259:string[])  [unwired: 1 out]
            n192 = Array Size(array=w259) -> (size(s)=→"总行数":i32)
            n193 = local write "校验码实际值"(w248) -> ()
            n194 = Add(x=w275, y=5) -> (x+y=w276:i32)
            n195 = Search/Split String(string=w268, search string/char (-)=")" ("搜索字符串/字符(-)")) -> ()  [unwired: 1 in, 3 out]
            n196 = String Subset(string=w265, offset (0)=45 ("偏移量(0)"), length (rest)=8 ("长度（剩余）")) -> ()  [unwired: 1 out]
            n197 = String Subset(string=w268, offset (0)=w276, length (rest)=32 ("长度（剩余）")) -> (substring=w266:string)
            n198 = Equal?(x=w266, y=w248) -> (x = y?=w273:bool)
            n199 = case shown="真" w273 {
              frame False {
                n200 = Build Array(cluster{u32, u32} {16711680, 0}) -> (w315:cluster{u32, u32}[])
                n201 = property on="MD5校验" class="Bool (严格)"("Colors [4]"=w315, "BoolText.Text"="失败" ("布尔文本.文本")) -> ()  [unwired: 2 in, 2 out]
              }
              frame True {
                n202 = Build Array(cluster{u32, u32} {6618880, 0}) -> (w318:cluster{u32, u32}[])
                n203 = property on="MD5校验" class="Bool (严格)"("Colors [4]"=w318, "BoolText.Text"="成功" ("布尔文本.文本")) -> ()  [unwired: 2 in, 2 out]
              }
            }
            n204 = local write "校验码期望值"(w266) -> ()
            n205 = for {
              tunnel: w259 -> [w296] mode=indexing
              shift-right: [w294] -> w249
              shift-left: u16 0 ("偏移量(0)") -> [w295]
              tunnel: [w288] -> w250 mode=indexing
              n206 = String Subset(string=w296, offset (0)=1 ("偏移量(0)"), length (rest)=1 ("长度（子字符串长度）")) -> (substring=w299:string)
              n207 = case shown="\"1\", 默认" w299 {
                tunnel: ["01" ("子字符串(\"\")") "02" ("子字符串(\"\")")] -> w300
                frame "1", Default {
                }
                frame "2" {
                }
              }
              n208 = String Subset(string=w296, offset (0)=2 ("偏移量(0)")) -> (substring=w302:string)  [unwired: 1 in]
              n209 = Concatenate Strings("FFFFFFFFFFFF" ("子字符串(\"\")"), w300, w302) -> (w288:string)
              n210 = String Subset(string=w288, offset (0)=12 ("偏移量(0)")) -> (substring=w286:string)  [unwired: 1 in]
              n211 = String Length(string=w286) -> (length=w293:i32)
              n212 = Divide(x=w293, y=2) -> (x/y=w291:dbl)
              n213 = for {
                N: w291 -> [_]
                tunnel: w286 -> [w311]
                shift-right: [w306] -> w289
                shift-left: u16 0 ("偏移量(0)") -> [w304]
                i -> [w310]
                w308 = 2 ("x")
                n214 = Multiply(x=w308, y=w310) -> (x*y=w309:i32)
                n215 = String Subset(string=w311, offset (0)=w309, length (rest)=w308) -> (substring=w307:string)
                n216 = call "ASCII_To_Hex.vi"("ASCII String"=w307) -> ("hex1"=w305:u8)  [unwired: 6 in, 4 out]
                n217 = Add(x=w304, y=w305) -> (x+y=w306:u16)
              }
              n218 = Add(x=w295, y=w289) -> (x+y=w294:u16)
            }
            n219 = local write "CRC16"(w249) -> ()
            n220 = local write "子数组"(w250) -> ()
          }
          frame True {
          }
        }
      }
      event "手动进入编程模式": Value Change {
        n221 = event-data() -> ("NewVal"=w320:bool)  [unwired: 1 in, 5 out]
        n222 = case shown="真" w320 {
          tunnel: w321 -> [_ w324]
          frame False {
          }
          frame True {
            n223 = Empty String/Path?(string/path="应用程序路径") -> (empty?=w322:bool)
            n224 = case shown="假" w322 {
              tunnel: w324 -> [w328 _]
              frame False {
                n225 = local write "update flag"(TRUE ("update flag")) -> ()
                n226 = Two Button Dialog(message="请确认需要下载的BMU编号正确！\nBMU正常上电！\n应用程序文件选择正确 !" ("消息")) -> (T button?=w327:bool)  [unwired: 2 in]
                n227 = case shown="真" w327 {
                  tunnel: w328 -> [_ w329]
                  frame False {
                  }
                  frame True {
                    n228 = stacked-sequence {
                      tunnel: w329 -> [_ _ _]
                      frame #0 {
                        n229 = disable-structure shown="启用" {
                          frame Enabled {
                            n230 = local read "CAN路数"() -> (w335:u32)
                            n231 = local read "设备索引"() -> (w336:u32)
                            n232 = local read "类型"() -> (w337:u32)
                            n233 = dll-call lib="F:/Bluewave New Energy/SVN_Work/AutoTest_TestStand/trunk/AutoTest_TestStand/Driver/ZlgCan/BHN01/AutoBurn/Settings/ControlCAN.dll" fn="VCI_ClearBuffer" label="VCI_Clearbuffer"(error in=errorcluster {"status"=FALSE, "code"=0, "source"=""} ("错误输入（无错误）"), "DeviceType"=w337, "DeviceInd"=w336, "CANInd"=w335) -> (error out=→"错误输出 3":errorcluster)  [unwired: 3 in, 4 out]
                          }
                          frame Disabled {
                          }
                        }
                        n234 = local write "boot模式应答...成功"(FALSE) -> ()
                        "boot模式应答计数" <- 0
                        "进入烧录" <- TRUE ("布尔")
                      }
                      frame #1 {
                        w343 = TRUE ("T1")
                        w342 = TRUE ("T1")
                        n235 = Concatenate Strings("" ("字符串"), "boot模式请求..." ("字符串"), "\n") -> (w341:string)
                        n236 = local write "Info："(w341) -> ()
                        n237 = local write "T2"(w342) -> ()
                        n238 = local write "T3"(w343) -> ()
                        n239 = local write "T1"(w342) -> ()
                        n240 = local write "T4"(w343) -> ()
                        n241 = local write "T5"(w343) -> ()
                        n242 = local write "T6"(w343) -> ()
                        n243 = local write "T7"(w343) -> ()
                        n244 = local write "T8"(u8 0 ("T8")) -> ()
                        n245 = local write "T9"(w343) -> ()
                      }
                      frame #2 {
                        n246 = local read "目标板类型"() -> (w346:enum16{"BCU/主板", "BMU/从板"})
                        n247 = case shown="\"BMU/从板\"" w346 {
                          tunnel: [u16 0 ("请选择板号") w359] -> w347
                          frame "BCU/主板", Default {
                          }
                          frame "BMU/从板" {
                            n248 = local read "请选择板号"() -> (w359:u16)
                          }
                        }
                        n249 = Tick Count (ms)() -> (millisecond timer value=→"start":u32)
                        n250 = Multiply(x=w347, y=u16 256) -> (x*y=w350:u16)
                        n251 = Add(x=u32 65681 ("ID"), y=w350) -> (x+y=w348:u32)
                        n252 = local read "VCI_CAN_OBJ_T"() -> (w352:T1)
                        n253 = case shown="1, 默认" w347 {
                          tunnel: [w364 w376] -> w356
                          tunnel: w352 -> [w363 w375]
                          tunnel: w348 -> [w361 w373]
                          frame 0 {
                            w360 = u8 170
                            w367 = u8 0 ("元素")
                            n254 = Bundle(cluster=w363, "ID"=w361, "TimeStamp"=u8 0 ("RemoteFlag"), "TimeFlag"=u8 1, "SendType"=u8 0 ("DataLen"), "RemoteFlag"=u8 0, "ExternFlag"=u8 1, "DataLen"=u8 8, u8 1 ("元素"), w360, w360, w360, w360, w367, w367, w367) -> (w364:T1)  [unwired: 3 in]
                          }
                          frame 1, Default {
                            w372 = u8 187
                            w379 = u8 0 ("元素")
                            n255 = Bundle(cluster=w375, "ID"=w373, "TimeStamp"=u8 0 ("RemoteFlag"), "TimeFlag"=u8 1, "SendType"=u8 0 ("DataLen"), "RemoteFlag"=u8 0, "ExternFlag"=u8 1, "DataLen"=u8 8, u8 1 ("元素"), w372, w372, w372, w372, w379, w379, w379) -> (w376:T1)  [unwired: 3 in]
                          }
                        }
                        n256 = local read "设备索引"() -> (w354:u32)
                        n257 = local read "CAN路数"() -> (w353:u32)
                        n258 = local read "类型"() -> (w355:u32)
                        n259 = dll-call lib="F:/Bluewave New Energy/SVN_Work/AutoTest_TestStand/trunk/AutoTest_TestStand/Driver/ZlgCan/BHN01/AutoBurn/Settings/ControlCAN.dll" fn="VCI_Transmit"("DeviceType"=w355, "DeviceInd"=w354, "CANInd"=w353, "pSend"=w356, "Len"=u32 1) -> ()  [unwired: 5 in, 6 out]
                      }
                    }
                  }
                }
              }
              frame True {
                n260 = One Button Dialog(message="请先选择应用程序路径" ("消息")) -> ()  [unwired: 1 in, 1 out]
              }
            }
          }
        }
      }
      event "开始监控 2": Value Change {
        n261 = event-data() -> ("NewVal"=w385:bool)  [unwired: 1 in, 5 out]
        n262 = local write "TEMP"(w385) -> ()
      }
      event Panel Close? {
        n263 = event-data() -> ()  [unwired: 1 in, 4 out]
        n264 = disable-structure shown="禁用" {
          frame Disabled {
            n265 = local read "设备索引"() -> (w389:u32)
            n266 = local read "CAN路数"() -> (w391:u32)
            n267 = local read "波特率"() -> (w390:T2)
            n268 = local read "滤波方式"() -> (w392:u8)
            n269 = local read "工作方式"() -> (w393:u8)
            n270 = local read "类型"() -> (w388:u32)
            n271 = call "CAN_Init.vi"("设备类型"=w388, "设备索引"=w389, "波特率"=w390, "CAN路数"=w391, "操作类型"=enum16{"初始化CAN", "关闭CAN"}."关闭CAN", 6:w392, 10:w393) -> (19:w387)  [unwired: 11 in, 1 out]
            n272 = flat-sequence {
              tunnel: w387 -> [_]
              frame #0 {
                n273 = Quit LabVIEW(quit? (T)=TRUE ("退出？(T)")) -> ()
              }
            }
          }
          frame Enabled {
          }
        }
        n274 = event-data("Discard?"=TRUE ("放弃？")) -> ()  [unwired: 1 in, 1 out]
      }
    }
    n275 = local read "退出？(T)"() -> (w44:bool)
  }
  n276 = while {
    tunnel: w25 -> [w402]
    tunnel: [w401] -> w9
    tunnel: "错误输入（无错误）" -> [w400]
    tunnel: [w399] -> w8
    tunnel: w24 -> [w398]
    stop <- w396 stop-if-true
    n277 = disable-structure shown="启用" {
      disable-tunnel: [w403 TRUE ("连接状态")] -> w397
      frame Disabled {
        n278 = local read "连接状态"() -> (w403:bool)
      }
      frame Enabled {
      }
    }
    n279 = case shown="真" w397 {
      tunnel: w402 -> [w408 w433]
      tunnel: [w408 w432] -> w401
      tunnel: w400 -> [w406 w431]
      tunnel: [w406 w430] -> w399
      tunnel: [w405 _] -> _
      tunnel: w398 -> [_ w418]
      frame False {
        n280 = disable-structure shown="禁用" {
          disable-tunnel: w406 -> [w410 w414]
          disable-tunnel: [w409 w414] -> w405
          frame Disabled {
            n281 = local read "设备索引"() -> (w412:u32)
            n282 = local read "CAN路数"() -> (w411:u32)
            n283 = local read "类型"() -> (w413:u32)
            n284 = dll-call lib="F:/Bluewave New Energy/SVN_Work/AutoTest_TestStand/trunk/AutoTest_TestStand/Driver/ZlgCan/BHN01/AutoBurn/Settings/ControlCAN.dll" fn="VCI_ClearBuffer" label="VCI_Clearbuffer"(error in=w410, "DeviceType"=w413, "DeviceInd"=w412, "CANInd"=w411) -> (error out=w409:errorcluster)  [unwired: 3 in, 4 out]
          }
          frame Enabled {
          }
        }
        n285 = Wait (ms)(milliseconds to wait=u32 50 ("等待时间（毫秒）")) -> ()  [unwired: 1 out]
      }
      frame True {
        (unwired) TRUE
        n286 = local read "CAN路数"() -> (w420:u32)
        n287 = local read "设备索引"() -> (w421:u32)
        n288 = local read "类型"() -> (w422:u32)
        n289 = dll-call lib="F:/Bluewave New Energy/SVN_Work/AutoTest_TestStand/trunk/AutoTest_TestStand/Driver/ZlgCan/BHN01/AutoBurn/Settings/ControlCAN.dll" fn="VCI_Receive"(error in=w431, "DeviceType"=w422, "DeviceInd"=w421, "CANInd"=w420, "pReceive"=w418, "Len"=u32 1, "WaitTime"=10) -> (error out=w425:errorcluster, "返回类型"=w426:u32, "pReceive"=w424:T1)  [unwired: 7 in, 1 out]
        "接收" <- w424
        n290 = Equal?(x=w426, y=1) -> (x = y?=w415:bool)
        n291 = Unbundle(w424) -> ("ID"=w416:u32, w419:u8)  [unwired: 16 out]
        n292 = Equal?(x=u32 4, y=w416) -> (x = y?=w417:bool)
        n293 = And(x=w417, y=w415) -> ()  [unwired: 1 out]
        n294 = case shown="真" w415 {
          tunnel: w433 -> [w435 w446]
          tunnel: [w435 w445] -> w432
          tunnel: w424 -> [_ w444]
          tunnel: w425 -> [w434 w443]
          tunnel: [w434 w442] -> w430
          tunnel: w419 -> [_ w439]
          tunnel: w422 -> [_ w438]
          tunnel: w421 -> [_ w437]
          tunnel: w420 -> [_ w436]
          frame False {
          }
          frame True {
            n295 = disable-structure shown="禁用" {
              disable-tunnel: w439 -> [w452 _]
              disable-tunnel: w438 -> [w450 _]
              disable-tunnel: w437 -> [w449 _]
              disable-tunnel: w436 -> [w448 _]
              frame Disabled {
                n296 = Equal?(x=w452, y=255) -> (x = y?=w447:bool)
                n297 = case shown="真" w447 {
                  tunnel: w450 -> [_ w457]
                  tunnel: w449 -> [_ w456]
                  tunnel: w448 -> [_ w455]
                  frame False {
                  }
                  frame True {
                    n298 = dll-call lib="F:/Bluewave New Energy/SVN_Work/AutoTest_TestStand/trunk/AutoTest_TestStand/Driver/ZlgCan/BHN01/AutoBurn/Settings/ControlCAN.dll" fn="VCI_Transmit"("DeviceType"=w457, "DeviceInd"=w456, "CANInd"=w455, "pSend"=T1 {"ID"=0, "TimeStamp"=0, "TimeFlag"=1, "SendType"=0, "RemoteFlag"=0, "ExternFlag"=0, "DataLen"=1, 1, 0, 0, 0, 0, 0, 0, 0, 0, 0, 0} ("输出簇 2"), "Len"=u32 1) -> ()  [unwired: 5 in, 6 out]
                  }
                }
              }
              frame Enabled {
              }
            }
            n299 = local read "CAN数据"() -> (w441:bool)
            n300 = Enqueue Element(queue=w446, element=w444, error in (no error)=w443) -> (queue out=w445:refnum<queue>, error out=w442:errorcluster)  [unwired: 1 in, 1 out]
            n301 = Not(x=w441) -> (.not. x?=w440:bool)
            n302 = local write "CAN数据"(w440) -> ()
          }
        }
      }
    }
    n303 = local read "退出？(T)"() -> (w396:bool)
  }
  n304 = stacked-sequence {
    tunnel: "错误输入（无错误）" -> [w478 w518 w629]
    frame #0 {
      w496 = "BURNRESULT" ("section")
      # "识别CAN卡，文件路径等"
      n305 = disable-structure shown="启用" {
        frame Enabled {
          w514 = u32 21 items=["PCI5121"=1, "PCI9810"=2, "USBCAN1"=3, "USBCAN2"=4, "PCI9820"=5, "CAN232"=6, "PCI5110"=7, "CANLite(mini)"=8, "ISA9620"=9, "ISA5420"=10, "PC104CAN"=11, "CANET"=17, "DNP9810"=13, "USBCAN-E-U"=20, "USBCAN-2E-U"=21] ("类型")
          w513 = u32 4 items=["PCI5121"=1, "PCI9810"=2, "USBCAN1"=3, "USBCAN2"=4, "PCI9820"=5, "CAN232"=6, "PCI5110"=7, "CANLite(mini)"=8, "ISA9620"=9, "ISA5420"=10, "PC104CAN"=11, "CANET"=17, "DNP9810"=13, "USBCAN-E-U"=20, "USBCAN-2E-U"=21] ("类型")
          n306 = Select(t=w513, s=FALSE, f=w514) -> (s? t:f=w515:u32)
          n307 = local write "类型"(w515) -> ()
        }
        frame Disabled {
        }
      }
      n308 = call <vilib>:"Open Config Data.vi"("error in (no error)"=w478, "configuration file path"=path "D:/BlueWay/configresult.ini") -> ("error out"=w494:errorcluster, "refnum"=w497:T4)  [unwired: 7 in, 1 out]
      n309 = call <vilib>:"Open Config Data.vi"("error in (no error)"=w478, "configuration file path"=path "D:/BlueWay/BMU从板号.ini") -> ("error out"=w484:errorcluster, "refnum"=w482:T4)  [unwired: 7 in, 1 out]
      n310 = call <vilib>:"Open Config Data.vi"("error in (no error)"=w478, "configuration file path"=path "D:/自动测试项目文件/ProjectSetting.ini") -> ("error out"=w485:errorcluster, "refnum"=w463:T4)  [unwired: 7 in, 1 out]
      n311 = call-poly <vilib>:"Write Key.vi"("section"=w496, "error in (no error)"=w494, "value"="FAIL" ("section"), "key"=w496, "refnum"=w497) -> ("error out"=w492:errorcluster, "refnum out"=w493:T4)  [unwired: 4 in, 1 out]
      n312 = call <vilib>:"Close Config Data.vi"("error in (no error)"=w492, "refnum"=w493) -> ()  [unwired: 8 in, 2 out]
      n313 = call-poly <vilib>:"Read Key.vi"("section"="BMUNO", "error in (no error)"=w484, "key"="BMUNO", "refnum"=w482) -> ("error out"=w470:errorcluster, "value"=w487:string, "refnum out"=w471:T4)  [unwired: 4 in, 1 out]
      n314 = disable-structure shown="禁用" {
        disable-tunnel: w487 -> [w517 _]
        frame Disabled {
          n315 = Decimal String To Number(string=w517) -> (number=w516:i32)  [unwired: 2 in, 1 out]
          n316 = local write "请选择板号"(w516) -> ()
        }
        frame Enabled {
        }
      }
      n317 = disable-structure shown="启用" {
        disable-tunnel: [w511 _] -> _
        disable-tunnel: w485 -> [w510 _]
        disable-tunnel: w463 -> [w509 _]
        frame Enabled {
          n318 = call-poly <vilib>:"Read Key.vi"("section"="PROJECT", "error in (no error)"=w510, "key"="内部CAN波特率", "refnum"=w509) -> ("value"=w508:string, "refnum out"=w511:T4)  [unwired: 4 in, 2 out]
          n319 = Equal?(x=w508, y="500K") -> (x = y?=w505:bool)
          n320 = Select(t=T2."500Kbps" ("波特率"), s=w505, f=T2."250Kbps" ("波特率")) -> (s? t:f=w501:T2)
          n321 = local write "波特率"(w501) -> ()
        }
        frame Disabled {
        }
      }
      n322 = Concatenate Strings("BMU" ("字符串"), w487) -> (w489:string)
      n323 = call-poly <vilib>:"Read Key.vi"("section"="PROJECT", "key"=w489, "refnum"=w463) -> ("value"=w490:string)  [unwired: 5 in, 3 out]
      n324 = call-poly <vilib>:"Read Key.vi"("section"="PROJECT", "key"="BCU应用程序", "refnum"=w463) -> ("value"=w465:string)  [unwired: 5 in, 3 out]
      n325 = call-poly <vilib>:"Read Key.vi"("section"="BMUTYPE", "error in (no error)"=w470, "key"="BMUTYPE", "refnum"=w471) -> ("error out"=w475:errorcluster, "value"=w476:string, "refnum out"=w474:T4)  [unwired: 4 in, 1 out]
      n326 = Build Path(base path=path "D:/自动测试项目文件" ("基路径"), name or relative path=w490) -> (appended path=w468:path)
      n327 = Build Path(base path=path "D:/自动测试项目文件" ("基路径"), name or relative path=w465) -> (appended path=w458:path)
      n328 = Equal?(x=w476, y="通用") -> (x = y?=w469:bool)
      n329 = call <vilib>:"Close Config Data.vi"("error in (no error)"=w475, "refnum"=w474) -> ()  [unwired: 8 in, 2 out]
      n330 = Select(t=path "D:/BlueWay/通用文件/TYXXXXSSXXXX.s19" ("基路径"), s=w469, f=w468) -> (s? t:f=w459:path)
      n331 = case shown="\"BCU/主板\", 默认" "板类型" {
        tunnel: [w499 w500] -> w460
        tunnel: w459 -> [_ w500]
        tunnel: w458 -> [w499 _]
        frame "BCU/主板", Default {
        }
        frame "BMU/从板" {
        }
      }
      n332 = local write "应用程序路径"(w460) -> ()
    }
    frame #1 {
      n333 = local read "应用程序路径"() -> (w519:path)
      n334 = Not A Number/Path/Refnum?(number/path/refnum=w519) -> (NaN/Path/Refnum?=w523:bool)
      n335 = Strip Path(path=w519) -> (name=w526:string)  [unwired: 1 out]
      n336 = String Subset(string=w526, offset (0)=6 ("偏移量(0)"), length (rest)=2 ("长度（剩余）")) -> (substring=w522:string)
      n337 = case shown="\"MS\"" w522 {
        tunnel: [TRUE ("y") FALSE ("y") FALSE ("y")] -> w525
        frame "假", Default {
          n338 = local read "Info："() -> (w528:string)
          n339 = Concatenate Strings(w528, "无法识别板类型！\n" ("字符串")) -> (w530:string)
          n340 = local write "Info："(w530) -> ()
        }
        frame "MS" {
          n341 = local read "Info："() -> (w532:string)
          n342 = local write "目标板类型"(enum16{"BCU/主板", "BMU/从板"}."BCU/主板" ("类型")) -> ()
          n343 = property on="请选择板号" class="Ring (严格)"("Visible"=FALSE ("可见")) -> ()  [unwired: 2 in, 2 out]
          n344 = Concatenate Strings(w532, "通过文件识别为主板！\n" ("字符串")) -> (w533:string)
          n345 = local write "Info："(w533) -> ()
        }
        frame "SS" {
          n346 = local read "Info："() -> (w538:string)
          n347 = local write "目标板类型"(enum16{"BCU/主板", "BMU/从板"}."BMU/从板" ("类型")) -> ()
          n348 = property on="请选择板号" class="Ring (严格)"("Visible"=TRUE ("可见")) -> ()  [unwired: 2 in, 2 out]
          n349 = Concatenate Strings(w538, "通过文件识别为从板！\n" ("字符串")) -> (w539:string)
          n350 = local write "Info："(w539) -> ()
        }
      }
      n351 = Or(x=w523, y=w525) -> (x .or. y?=w524:bool)
      n352 = case shown="真" w524 {
        tunnel: w519 -> [w579 _]
        tunnel: w518 -> [w543 _]
        frame False {
          n353 = Path To String(path=w579) -> (string=w554:string)
          n354 = local read "Info："() -> (w550:string)
          n355 = String Subset(string=w554, offset (0)=6 ("偏移量(0)"), length (rest)=2 ("长度（剩余）")) -> (substring=w551:string)
          n356 = call-poly <vilib>:"Read From Spreadsheet File.vi"("file path (dialog if empty)"=w579) -> ("all rows"=w581:string[][])  [unwired: 6 in, 4 out]
          n357 = call <vilib>:"Space Constant.vi"() -> ("String"=w577:string)
          n358 = Search and Replace String(replace all?=TRUE ("替换全部？(F)"), input string=w554, search string=w577, replace string="" ("替换字符串(\"\")")) -> (result string=w564:string)  [unwired: 4 in, 3 out]
          n359 = case shown="\"真\"" w551 {
            frame "假", Default {
            }
            frame "真" {
            }
          }
          n360 = Concatenate Strings(w550, "文件加载成功！\n" ("字符串")) -> (w548:string)
          n361 = Index Array(array=w581, index (col)=0 ("禁用的索引 (列)")) -> (element=w568:string[])  [unwired: 1 in]
          n362 = Search/Split String(string=w564, search string/char (-)="(MD5=" ("搜索字符串/字符(-)")) -> (match + rest of string=w561:string, offset of match=w571:i32)  [unwired: 1 in, 1 out]
          n363 = local write "Info："(w548) -> ()
          n364 = Delete From Array(array=w568, length=1 ("长度"), index=0 ("索引")) -> (array with subset deleted=w560:string[])  [unwired: 1 out]
          n365 = call <vilib>:"MD5Checksum File.vi"("error in (no error)"=w543, "Path"=w579) -> ("MD5 message-digest"=w545:string)  [unwired: 8 in, 1 out]
          n366 = Array Size(array=w560) -> (size(s)=w558:i32)
          n367 = Decrement(x=w558) -> (x-1=w557:i32)
          n368 = Delete From Array(array=w560, length=1 ("长度"), index=w557) -> (array with subset deleted=w556:string[])  [unwired: 1 out]
          n369 = Array Size(array=w556) -> (size(s)=w544:i32)
          n370 = local write "校验码实际值"(w545) -> ()
          n371 = Add(x=w571, y=5) -> (x+y=w572:i32)
          n372 = Search/Split String(string=w564, search string/char (-)=")" ("搜索字符串/字符(-)")) -> ()  [unwired: 1 in, 3 out]
          n373 = String Subset(string=w561, offset (0)=45 ("偏移量(0)"), length (rest)=8 ("长度（剩余）")) -> ()  [unwired: 1 out]
          n374 = local write "总行数"(w544) -> ()
          n375 = String Subset(string=w564, offset (0)=w572, length (rest)=32 ("长度（剩余）")) -> (substring=w562:string)
          n376 = Equal?(x=w562, y=w545) -> (x = y?=w569:bool)
          n377 = case shown="真" w569 {
            frame False {
              n378 = Build Array(cluster{u32, u32} {16711680, 0}) -> (w611:cluster{u32, u32}[])
              n379 = property on="MD5校验" class="Bool (严格)"("Colors [4]"=w611, "BoolText.Text"="失败" ("布尔文本.文本")) -> ()  [unwired: 2 in, 2 out]
            }
            frame True {
              n380 = Build Array(cluster{u32, u32} {6618880, 0}) -> (w614:cluster{u32, u32}[])
              n381 = property on="MD5校验" class="Bool (严格)"("Colors [4]"=w614, "BoolText.Text"="成功" ("布尔文本.文本")) -> ()  [unwired: 2 in, 2 out]
            }
          }
          n382 = local write "校验码期望值"(w562) -> ()
          n383 = for {
            tunnel: w556 -> [w592] mode=indexing
            shift-right: [w590] -> w546
            shift-left: u16 0 ("偏移量(0)") -> [w591]
            tunnel: [w584] -> w547 mode=indexing
            n384 = String Subset(string=w592, offset (0)=1 ("偏移量(0)"), length (rest)=1 ("长度（子字符串长度）")) -> (substring=w595:string)
            n385 = case shown="\"1\", 默认" w595 {
              tunnel: ["01" ("子字符串(\"\")") "02" ("子字符串(\"\")")] -> w596
              frame "1", Default {
              }
              frame "2" {
              }
            }
            n386 = String Subset(string=w592, offset (0)=2 ("偏移量(0)")) -> (substring=w598:string)  [unwired: 1 in]
            n387 = Concatenate Strings("FFFFFFFFFFFF" ("子字符串(\"\")"), w596, w598) -> (w584:string)
            n388 = String Subset(string=w584, offset (0)=12 ("偏移量(0)")) -> (substring=w582:string)  [unwired: 1 in]
            n389 = String Length(string=w582) -> (length=w589:i32)
            n390 = Divide(x=w589, y=2) -> (x/y=w587:dbl)
            n391 = for {
              N: w587 -> [_]
              tunnel: w582 -> [w607]
              shift-right: [w602] -> w585
              shift-left: u16 0 ("偏移量(0)") -> [w600]
              i -> [w606]
              w604 = 2 ("x")
              n392 = Multiply(x=w604, y=w606) -> (x*y=w605:i32)
              n393 = String Subset(string=w607, offset (0)=w605, length (rest)=w604) -> (substring=w603:string)
              n394 = call "ASCII_To_Hex.vi"("ASCII String"=w603) -> ("hex1"=w601:u8)  [unwired: 6 in, 4 out]
              n395 = Add(x=w600, y=w601) -> (x+y=w602:u16)
            }
            n396 = Add(x=w591, y=w585) -> (x+y=w590:u16)
          }
          n397 = local write "CRC16"(w546) -> ()
          n398 = local write "子数组"(w547) -> ()
        }
        frame True {
          n399 = flat-sequence {
            frame #0 {
              n400 = local read "Info："() -> (w617:string)
              n401 = Concatenate Strings(w617, "文件加载错误！\n" ("字符串")) -> (w616:string)
              n402 = local write "Info："(w616) -> ()
            }
            frame #1 {
              n403 = Wait (ms)(milliseconds to wait=u32 2000 ("等待时间（毫秒）")) -> ()  [unwired: 1 out]
            }
            frame #2 {
              n404 = disable-structure shown="禁用" {
                frame Disabled {
                  n405 = local read "设备索引"() -> (w621:u32)
                  n406 = local read "CAN路数"() -> (w623:u32)
                  n407 = local read "波特率"() -> (w622:T2)
                  n408 = local read "滤波方式"() -> (w624:u8)
                  n409 = local read "工作方式"() -> (w625:u8)
                  n410 = local read "类型"() -> (w620:u32)
                  n411 = call "CAN_Init.vi"("设备类型"=w620, "设备索引"=w621, "波特率"=w622, "CAN路数"=w623, "操作类型"=enum16{"初始化CAN", "关闭CAN"}."关闭CAN", 6:w624, 10:w625) -> ()  [unwired: 12 in, 1 out]
                }
                frame Enabled {
                }
              }
            }
            frame #3 {
              n412 = Quit LabVIEW(quit? (T)=TRUE ("退出？(T)")) -> ()
            }
          }
        }
      }
    }
    frame #2 {
      w633 = "" ("布尔文本.文本")
      w634 = cluster{u32, u32}[] [{0, 0}] ("颜色[4]")
      w635 = FALSE
      n413 = local write "update flag"(TRUE ("update flag")) -> ()
      n414 = disable-structure shown="禁用" {
        disable-tunnel: [_ TRUE ("连接状态")] -> w631
        disable-tunnel: w629 -> [_ _]
        disable-tunnel: [errorcluster {"status"=FALSE, "code"=0, "source"=""} ("error out") _] -> w628
        frame Disabled {
        }
        frame Enabled {
        }
      }
      n415 = property on="烧录结果" class="Bool (严格)"("Colors [4]"=w634, "BoolText.Text"=w633) -> ()  [unwired: 2 in, 2 out]
      n416 = property on="校验" class="Bool (严格)"("Colors [4]"=w634, "BoolText.Text"=w633) -> ()  [unwired: 2 in, 2 out]
      n417 = local write "擦除完成"(w635) -> ()
      n418 = local write "进入烧录模式"(w635) -> ()
      n419 = local write "烧录结果"(w635) -> ()
      n420 = local write "进度"(u8 0 ("进度")) -> ()
      n421 = local write "CAN状态"(w631) -> ()
      n422 = local write "连接状态"(w631) -> ()
      n423 = local write "Monitor_flag"(FALSE ("Monitor_flag")) -> ()
      n424 = case shown="真" w631 {
        tunnel: w629 -> [w639 _]
        tunnel: w628 -> [_ _]
        frame True {
          n425 = local read "Info："() -> (w640:string)
          n426 = stacked-sequence {
            tunnel: w639 -> [w649 _ _]
            tunnel: [w648 _ _] -> _
            frame #0 {
              n427 = disable-structure shown="启用" {
                disable-tunnel: w649 -> [w652 _]
                disable-tunnel: [w651 _] -> w648
                frame Enabled {
                  n428 = local read "CAN路数"() -> (w653:u32)
                  n429 = local read "设备索引"() -> (w654:u32)
                  n430 = local read "类型"() -> (w655:u32)
                  n431 = dll-call lib="F:/Bluewave New Energy/SVN_Work/AutoTest_TestStand/trunk/AutoTest_TestStand/Driver/ZlgCan/BHN01/AutoBurn/Settings/ControlCAN.dll" fn="VCI_ClearBuffer" label="VCI_Clearbuffer"(error in=w652, "DeviceType"=w655, "DeviceInd"=w654, "CANInd"=w653) -> (error out=w651:errorcluster)  [unwired: 3 in, 4 out]
                }
                frame Disabled {
                }
              }
              n432 = local write "boot模式应答...成功"(FALSE) -> ()
              n433 = local write "开始下载数据"(FALSE ("开始下载数据")) -> ()
              n434 = local write "进入烧录"(TRUE ("布尔")) -> ()
              n435 = local write "开始下载数据"(u32 0 ("开始下载数据")) -> ()
              n436 = local write "boot模式应答计数"(0 ("boot模式应答计数")) -> ()
            }
            frame #1 {
              w661 = TRUE ("T1")
              w660 = TRUE ("T1")
              n437 = local read "Info："() -> (w656:string)
              n438 = Concatenate Strings(w656, "boot模式请求..." ("字符串"), "\n") -> (w659:string)
              n439 = local write "Info："(w659) -> ()
              n440 = local write "T2"(w660) -> ()
              n441 = local write "T3"(w661) -> ()
              n442 = local write "T1"(w660) -> ()
              n443 = local write "T4"(w661) -> ()
              n444 = local write "T5"(w661) -> ()
              n445 = local write "T6"(w661) -> ()
              n446 = local write "T7"(w661) -> ()
              n447 = local write "T8"(u8 0 ("T8")) -> ()
              n448 = local write "T9"(w661) -> ()
            }
            frame #2 {
              n449 = local read "目标板类型"() -> (w664:enum16{"BCU/主板", "BMU/从板"})
              n450 = Tick Count (ms)() -> (millisecond timer value=w663:u32)
              n451 = case shown="\"BCU/主板\", 默认" w664 {
                tunnel: [u16 0 ("请选择板号") w677] -> w665
                frame "BCU/主板", Default {
                }
                frame "BMU/从板" {
                  n452 = local read "请选择板号"() -> (w677:u16)
                }
              }
              n453 = local write "start"(w663) -> ()
              n454 = Multiply(x=w665, y=u16 256) -> (x*y=w668:u16)
              n455 = Add(x=u32 65681 ("ID"), y=w668) -> (x+y=w666:u32)
              n456 = local read "VCI_CAN_OBJ_T"() -> (w670:T1)
              n457 = case shown="1, 默认" w665 {
                tunnel: [w682 w694] -> w674
                tunnel: w670 -> [w681 w693]
                tunnel: w666 -> [w679 w691]
                frame 0 {
                  w678 = u8 170
                  w685 = u8 0 ("元素")
                  n458 = Bundle(cluster=w681, "ID"=w679, "TimeStamp"=u8 0 ("RemoteFlag"), "TimeFlag"=u8 1, "SendType"=u8 0 ("DataLen"), "RemoteFlag"=u8 0, "ExternFlag"=u8 1, "DataLen"=u8 8, u8 1 ("元素"), w678, w678, w678, w678, w685, w685, w685) -> (w682:T1)  [unwired: 3 in]
                }
                frame 1, Default {
                  w690 = u8 187
                  w697 = u8 0 ("元素")
                  n459 = Bundle(cluster=w693, "ID"=w691, "TimeStamp"=u8 0 ("RemoteFlag"), "TimeFlag"=u8 1, "SendType"=u8 0 ("DataLen"), "RemoteFlag"=u8 0, "ExternFlag"=u8 1, "DataLen"=u8 8, u8 1 ("元素"), w690, w690, w690, w690, w697, w697, w697) -> (w694:T1)  [unwired: 3 in]
                }
              }
              n460 = local read "设备索引"() -> (w672:u32)
              n461 = local read "CAN路数"() -> (w671:u32)
              n462 = local read "类型"() -> (w673:u32)
              n463 = dll-call lib="F:/Bluewave New Energy/SVN_Work/AutoTest_TestStand/trunk/AutoTest_TestStand/Driver/ZlgCan/BHN01/AutoBurn/Settings/ControlCAN.dll" fn="VCI_Transmit"("DeviceType"=w673, "DeviceInd"=w672, "CANInd"=w671, "pSend"=w674, "Len"=u32 1) -> ()  [unwired: 5 in, 6 out]
            }
          }
          n464 = Concatenate Strings(w640, "启动CAN成功.." ("字符串"), "\n") -> (w643:string)
          n465 = local write "Info："(w643) -> ()
        }
        frame False {
          n466 = stacked-sequence {
            frame #0 {
              n467 = local read "Info："() -> (w702:string)
              n468 = Concatenate Strings(w702, "启动CAN失败.." ("字符串"), "\n") -> (w705:string)
              n469 = local write "Info："(w705) -> ()
            }
            frame #1 {
              n470 = disable-structure shown="禁用" {
                frame Disabled {
                  n471 = local read "设备索引"() -> (w708:u32)
                  n472 = local read "CAN路数"() -> (w710:u32)
                  n473 = local read "波特率"() -> (w709:T2)
                  n474 = local read "滤波方式"() -> (w711:u8)
                  n475 = local read "工作方式"() -> (w712:u8)
                  n476 = local read "类型"() -> (w707:u32)
                  n477 = call "CAN_Init.vi"("设备类型"=w707, "设备索引"=w708, "波特率"=w709, "CAN路数"=w710, "操作类型"=enum16{"初始化CAN", "关闭CAN"}."关闭CAN", 6:w711, 10:w712) -> ()  [unwired: 12 in, 1 out]
                }
                frame Enabled {
                }
              }
              n478 = Wait (ms)(milliseconds to wait=u32 2000 ("等待时间（毫秒）")) -> ()  [unwired: 1 out]
            }
            frame #2 {
              n479 = Quit LabVIEW(quit? (T)=TRUE ("退出？(T)")) -> ()
            }
          }
        }
      }
    }
  }
  n480 = while {
    tunnel: w25 -> [w721]
    shift-right: [w724] -> _
    shift-left: w38 -> [w725]
    shift-right: [w722] -> _
    shift-left: "" -> [w723]
    tunnel: w12 -> [w720]
    stop <- w715 stop-if-true
    n481 = local read "update flag"() -> (w717:bool)
    n482 = Dequeue Element(queue=w721, timeout in ms (-1)=100 ("超时毫秒(-1)"), error in (no error)=w720) -> (element=w718:T1, error out=w719:errorcluster)  [unwired: 2 out]
    n483 = case shown="假" w717 {
      tunnel: w725 -> [_ w743]
      tunnel: [_ w742] -> w724
      tunnel: w723 -> [_ w741]
      tunnel: [_ w740] -> w722
      tunnel: w721 -> [_ w738]
      tunnel: w719 -> [_ w737]
      tunnel: w718 -> [_ w736]
      frame False {
      }
      frame True {
        n484 = local read "VCI_CAN_OBJ_T"() -> (w746:T1)
        n485 = local read "CAN路数"() -> (w744:u32)
        n486 = Unbundle(w736) -> ("ID"=w735:u32, w734:u8, w733:u8, w732:u8, w731:u8, w730:u8, w729:u8, w728:u8, w727:u8)  [unwired: 9 out]
        n487 = local read "类型"() -> (w745:u32)
        n488 = local read "设备索引"() -> (w726:u32)
        n489 = case shown="FC" w735 {
          selector: w735 -> [_ w942 w1025 w1082 w1271 _ _ _ _ w2003]
          tunnel: w736 -> [_ _ _ _ _ _ _ _ _ _]
          tunnel: w746 -> [w760 _ _ w1086 w1275 w1485 w1550 _ w1786 _]
          tunnel: w745 -> [w759 _ _ w1085 w1274 w1484 w1552 w1680 w1794 _]
          tunnel: w726 -> [w758 _ _ w1084 w1273 w1483 w1551 w1679 w1793 _]
          tunnel: w744 -> [w757 _ _ w1083 w1272 w1482 w1549 w1678 w1792 _]
          tunnel: w743 -> [w756 _ _ _ _ w1481 w1554 w1677 w1788 w2005]
          tunnel: [w756 _ _ _ _ w1481 w1553 w1677 w1789 w2005] -> w742
          tunnel: w741 -> [w755 _ _ _ _ w1480 w1548 w1682 w1790 w2004]
          tunnel: [w755 _ _ _ _ w1480 w1547 w1681 w1791 w2004] -> w740
          tunnel: "板类型" -> [_ _ _ _ _ _ w1546 w1676 w1787 _]
          tunnel: w738 -> [_ _ _ _ _ w1479 w1545 w1675 w1785 _]
          tunnel: w737 -> [_ _ _ _ _ _ _ _ _ _]
          tunnel: w736 -> [_ _ _ _ _ _ _ w1666 _ _]
          tunnel: w736 -> [_ _ _ _ _ _ _ _ w1784 _]
          tunnel: w734 -> [w754 w945 w1027 w1089 _ _ _ _ _ _]
          tunnel: w733 -> [w753 w940 _ _ _ _ _ _ _ _]
          tunnel: w732 -> [w752 w939 _ _ w1269 _ _ _ _ _]
          tunnel: w731 -> [w751 w938 _ _ _ _ _ _ _ _]
          tunnel: w730 -> [w750 w937 _ _ _ _ _ _ _ _]
          tunnel: w729 -> [w749 _ _ _ _ _ _ _ _ _]
          tunnel: w728 -> [w748 _ _ _ _ _ _ _ _ w2002]
          tunnel: w727 -> [w747 _ _ _ _ _ _ _ _ w2001]
          frame 4 {
            (unwired) TRUE
            n490 = disable-structure shown="禁用" {
              disable-tunnel: w760 -> [w772 _]
              disable-tunnel: w759 -> [w771 _]
              disable-tunnel: w758 -> [w770 _]
              disable-tunnel: w757 -> [w769 _]
              disable-tunnel: w754 -> [w768 _]
              disable-tunnel: w753 -> [w767 _]
              disable-tunnel: w752 -> [w766 _]
              disable-tunnel: w751 -> [w765 _]
              disable-tunnel: w750 -> [w764 _]
              disable-tunnel: w749 -> [w763 _]
              disable-tunnel: w748 -> [w762 _]
              disable-tunnel: w747 -> [w761 _]
              frame Disabled {
                n491 = stacked-sequence {
                  tunnel: w772 -> [w797]
                  tunnel: w771 -> [w796]
                  tunnel: w770 -> [w795]
                  tunnel: w769 -> [w794]
                  tunnel: w768 -> [w793]
                  tunnel: w767 -> [w792]
                  tunnel: w766 -> [w791]
                  tunnel: w765 -> [w790]
                  tunnel: w764 -> [w789]
                  tunnel: w763 -> [w788]
                  tunnel: w762 -> [w787]
                  tunnel: w761 -> [w786]
                  frame #0 {
                    n492 = Equal?(x=w793, y=u8 252) -> (x = y?=w777:bool)
                    n493 = Equal?(x=w792, y=u8 7) -> (x = y?=w776:bool)
                    n494 = Equal?(x=w791, y=u8 3) -> (x = y?=w775:bool)
                    n495 = Equal?(x=w790, y=u8 255) -> (x = y?=w774:bool)
                    n496 = Equal?(x=w788, y=u8 0) -> ()  [unwired: 1 out]
                    n497 = Equal?(x=w786, y=u8 1) -> ()  [unwired: 1 out]
                    n498 = Equal?(x=w789, y=u8 0) -> ()  [unwired: 1 out]
                    n499 = Equal?(x=w787, y=u8 0) -> ()  [unwired: 1 out]
                    n500 = Compound Arithmetic op=AND(w777, w776, w775, w774) -> (w773:bool)
                    n501 = case shown="真" w773 {
                      tunnel: w797 -> [_ w805]
                      tunnel: w796 -> [_ w804]
                      tunnel: w795 -> [_ w803]
                      tunnel: w794 -> [_ w802]
                      frame False {
                      }
                      frame True {
                        n502 = local read "T8"() -> (w801:u8)
                        n503 = Increment(x=w801) -> (x+1=w800:u8)
                        n504 = Greater Or Equal?(x=w800, y=u8 10) -> (x >= y?=w798:bool)
                        n505 = local write "T8"(w800) -> ()
                        n506 = case shown="真" w798 {
                          tunnel: w805 -> [_ w815]
                          tunnel: w804 -> [_ w814]
                          tunnel: w803 -> [_ w813]
                          tunnel: w802 -> [_ w812]
                          frame False {
                          }
                          frame True {
                            n507 = local read "子数组"() -> (w811:string[])
                            n508 = local read "Info："() -> (w807:string)
                            n509 = Array Size(array=w811) -> (size(s)=w810:i32)
                            n510 = while {
                              tunnel: w815 -> [w826]
                              tunnel: w814 -> [w825]
                              tunnel: w813 -> [w824]
                              tunnel: w812 -> [w823]
                              tunnel: w811 -> [w822] mode=indexing
                              tunnel: w810 -> [w819]
                              i -> [w820]
                              stop <- w818 stop-if-true
                              n511 = while {
                                tunnel: w826 -> [w842]
                                tunnel: w825 -> [w841]
                                tunnel: w824 -> [w840]
                                tunnel: w823 -> [w839]
                                shift-right: [w834] -> _
                                shift-left: w822 -> [w835]
                                tunnel: w819 -> [w832]
                                tunnel: w820 -> [w828]
                                stop <- w827 stop-if-true
                                n512 = String Length(string=w835) -> (length=w833:i32)
                                n513 = Greater Or Equal?(x=w833, y=8) -> (x >= y?=w836:bool)
                                n514 = case shown="假" w836 {
                                tunnel: w842 -> [w870 w880]
                                tunnel: w841 -> [w869 w879]
                                tunnel: w840 -> [w868 w878]
                                tunnel: w839 -> [w867 w877]
                                tunnel: w835 -> [w856 w876]
                                tunnel: [w844 w875] -> w834
                                tunnel: [FALSE TRUE] -> w827
                                tunnel: w833 -> [_ w873]
                                tunnel: w833 -> [_ w871]
                                frame True {
                                w863 = u8 0 ("元素")
                                n515 = String Subset(string=w856, offset (0)=8 ("偏移量(0)")) -> (substring=w844:string)  [unwired: 1 in]
                                n516 = String Subset(string=w856, length (rest)=8 ("长度（剩余）")) -> (substring=w854:string)  [unwired: 1 in]
                                n517 = String To Byte Array(string=w854) -> (unsigned byte array=w853:u8[])
                                n518 = Index Array(array=w853) -> (element #1=w852:u8, element #2=w851:u8, element #3=w850:u8, element #4=w849:u8, element #5=w848:u8, element #6=w847:u8, element #7=w846:u8, element #8=w845:u8)  [unwired: 8 in]
                                n519 = Bundle(cluster=w870, "ID"=u32 5, "TimeStamp"=u8 0 ("RemoteFlag"), "TimeFlag"=u8 1, "SendType"=u8 0 ("DataLen"), "RemoteFlag"=u8 0, "DataLen"=u8 8, w852, w851, w850, w849, w848, w847, w846, w845, w863, w863, w863) -> (w858:T1)  [unwired: 1 in]
                                n520 = dll-call lib="F:/Bluewave New Energy/SVN_Work/AutoTest_TestStand/trunk/AutoTest_TestStand/Driver/ZlgCan/BHN01/AutoBurn/Settings/ControlCAN.dll" fn="VCI_Transmit"("DeviceType"=w869, "DeviceInd"=w868, "CANInd"=w867, "pSend"=w858, "Len"=u32 1) -> ()  [unwired: 5 in, 6 out]
                                }
                                frame False {
                                n521 = Greater Than 0?(x=w873) -> (x > 0?=w872:bool)
                                n522 = case shown="真" w872 {
                                tunnel: w880 -> [w907 w914]
                                tunnel: w879 -> [w906 w913]
                                tunnel: w878 -> [w905 w912]
                                tunnel: w877 -> [w904 w911]
                                tunnel: w876 -> [w893 _]
                                tunnel: [w882 _] -> w875
                                tunnel: w871 -> [_ w909]
                                frame True {
                                w900 = u8 0 ("元素")
                                n523 = String Subset(string=w893, offset (0)=8 ("偏移量(0)")) -> (substring=w882:string)  [unwired: 1 in]
                                n524 = String Subset(string=w893, length (rest)=8 ("长度（剩余）")) -> (substring=w892:string)  [unwired: 1 in]
                                n525 = String To Byte Array(string=w892) -> (unsigned byte array=w891:u8[])
                                n526 = Index Array(array=w891) -> (element #1=w890:u8, element #2=w889:u8, element #3=w888:u8, element #4=w887:u8, element #5=w886:u8, element #6=w885:u8, element #7=w884:u8, element #8=w883:u8)  [unwired: 8 in]
                                n527 = Bundle(cluster=w907, "ID"=u32 5, "TimeStamp"=u8 0 ("RemoteFlag"), "TimeFlag"=u8 1, "SendType"=u8 0 ("DataLen"), "RemoteFlag"=u8 0, "DataLen"=u8 8, w890, w889, w888, w887, w886, w885, w884, w883, w900, w900, w900) -> (w895:T1)  [unwired: 1 in]
                                n528 = dll-call lib="F:/Bluewave New Energy/SVN_Work/AutoTest_TestStand/trunk/AutoTest_TestStand/Driver/ZlgCan/BHN01/AutoBurn/Settings/ControlCAN.dll" fn="VCI_Transmit"("DeviceType"=w906, "DeviceInd"=w905, "CANInd"=w904, "pSend"=w895, "Len"=u32 1) -> ()  [unwired: 5 in, 6 out]
                                }
                                frame False {
                                n529 = Quotient & Remainder(x=w909, y=8) -> (x-y*floor(x/y)=w908:i32)  [unwired: 1 out]
                                n530 = case shown="0" w908 {
                                tunnel: w914 -> [w936 _]
                                tunnel: w913 -> [w935 _]
                                tunnel: w912 -> [w934 _]
                                tunnel: w911 -> [w933 _]
                                frame 0 {
                                w929 = u8 0 ("元素")
                                n531 = Index Array(array=u8[] [0, 0, 0, 0, 0, 0, 0, 0] ("数组")) -> (element #1=w923:u8, element #2=w922:u8, element #3=w921:u8, element #4=w920:u8, element #5=w919:u8, element #6=w918:u8, element #7=w917:u8, element #8=w916:u8)  [unwired: 8 in]
                                n532 = Bundle(cluster=w936, "ID"=u32 5, "TimeStamp"=u8 0 ("RemoteFlag"), "TimeFlag"=u8 1, "SendType"=u8 0 ("DataLen"), "RemoteFlag"=u8 0, "DataLen"=u8 8, w923, w922, w921, w920, w919, w918, w917, w916, w929, w929, w929) -> (w924:T1)  [unwired: 1 in]
                                n533 = dll-call lib="F:/Bluewave New Energy/SVN_Work/AutoTest_TestStand/trunk/AutoTest_TestStand/Driver/ZlgCan/BHN01/AutoBurn/Settings/ControlCAN.dll" fn="VCI_Transmit"("DeviceType"=w935, "DeviceInd"=w934, "CANInd"=w933, "pSend"=w924, "Len"=u32 1) -> ()  [unwired: 5 in, 6 out]
                                }
                                frame 1, Default {
                                }
                                }
                                }
                                }
                                }
                                }
                                n534 = Divide(x=w828, y=w832) -> (x/y=w831:dbl)
                                n535 = Multiply(x=w831, y=100.0) -> (x*y=w829:dbl)
                                n536 = local write "进度"(w829) -> ()
                                n537 = Wait (ms)(milliseconds to wait=u32 5 ("等待时间（毫秒）")) -> ()  [unwired: 1 out]
                              }
                              n538 = Equal?(x=w820, y=w819) -> (x = y?=w816:bool)
                              n539 = local read "连接状态"() -> (w821:bool)
                              n540 = Not(x=w821) -> (.not. x?=w817:bool)
                              n541 = Or(x=w816, y=w817) -> (x .or. y?=w818:bool)
                            }
                            n542 = Concatenate Strings(w807, "程序下载中.." ("字符串"), "\n") -> (w806:string)
                            n543 = local write "Info："(w806) -> ()
                          }
                        }
                      }
                    }
                  }
                }
              }
              frame Enabled {
              }
            }
          }
          frame 102656..102688, 102911 {
            n544 = To Unsigned Byte Integer(number=w942) -> (unsigned 8bit integer=w941:u8)
            n545 = Equal?(x=w945, y=u8 85) -> (x = y?=w944:bool)
            n546 = case shown="假" w944 {
              tunnel: w941 -> [_ w978]
              tunnel: w940 -> [_ w975]
              tunnel: w939 -> [_ w973]
              tunnel: w938 -> [_ w974]
              tunnel: w937 -> [_ w972]
              frame False {
                n547 = local write "update flag"(FALSE ("update flag")) -> ()
                n548 = disable-structure shown="禁用" {
                  frame Disabled {
                    n549 = flat-sequence {
                      frame #0 {
                        n550 = local read "设备索引"() -> (w959:u32)
                        n551 = local read "CAN路数"() -> (w957:u32)
                        n552 = local read "波特率"() -> (w958:T2)
                        n553 = local read "滤波方式"() -> (w956:u8)
                        n554 = local read "工作方式"() -> (w955:u8)
                        n555 = local read "类型"() -> (w960:u32)
                        n556 = call "CAN_Init.vi"("设备类型"=w960, "设备索引"=w959, "波特率"=w958, "CAN路数"=w957, "操作类型"=enum16{"初始化CAN", "关闭CAN"}."关闭CAN", 6:w956, 10:w955) -> ()  [unwired: 12 in, 1 out]
                        n557 = Wait (ms)(milliseconds to wait=u32 2000 ("等待时间（毫秒）")) -> ()  [unwired: 1 out]
                      }
                      frame #1 {
                        n558 = Quit LabVIEW(quit? (T)=TRUE ("退出？(T)")) -> ()
                      }
                    }
                  }
                  frame Enabled {
                  }
                }
                n559 = local read "Info："() -> (w949:string)
                n560 = One Button Dialog(message="程序下载错误，请断电重试！" ("消息")) -> ()  [unwired: 1 in, 1 out]
                n561 = Concatenate Strings(w949, "boot模式应答...失败" ("字符串"), "\n") -> (w952:string)
                n562 = local write "Info："(w952) -> ()
                n563 = local write "退出？(T)"(TRUE ("退出？(T)")) -> ()
              }
              frame True {
                n564 = Join Numbers(hi=w975, lo=w974) -> ((hi.lo)=w971:u16)
                n565 = Join Numbers(hi=w972, lo=w973) -> ((hi.lo)=w970:u16)
                n566 = Join Numbers(hi=w971, lo=w970) -> ((hi.lo)=w969:u32)
                n567 = Not(x=w969) -> (.not. x?=w968:u32)
                "Random" <- w968
                n568 = Split Number(x=w968) -> (hi(x)=w967:u16, lo(x)=w966:u16)
                n569 = Split Number(x=w967) -> (hi(x)=w965:u8, lo(x)=w964:u8)
                n570 = Split Number(x=w966) -> (hi(x)=w963:u8, lo(x)=w962:u8)
                n571 = stacked-sequence {
                  tunnel: w978 -> [_ w999]
                  tunnel: w965 -> [_ w994]
                  tunnel: w964 -> [_ w993]
                  tunnel: w963 -> [_ w992]
                  tunnel: w962 -> [_ w991]
                  frame #0 {
                    n572 = disable-structure shown="启用" {
                      frame Enabled {
                        n573 = local read "CAN路数"() -> (w986:u32)
                        n574 = local read "设备索引"() -> (w987:u32)
                        n575 = local read "类型"() -> (w988:u32)
                        n576 = dll-call lib="F:/Bluewave New Energy/SVN_Work/AutoTest_TestStand/trunk/AutoTest_TestStand/Driver/ZlgCan/BHN01/AutoBurn/Settings/ControlCAN.dll" fn="VCI_ClearBuffer" label="VCI_Clearbuffer"(error in=errorcluster {"status"=FALSE, "code"=0, "source"=""} ("错误输入（无错误）"), "DeviceType"=w988, "DeviceInd"=w987, "CANInd"=w986) -> (error out=→"错误输出 12":errorcluster)  [unwired: 3 in, 4 out]
                      }
                      frame Disabled {
                      }
                    }
                    n577 = Wait (ms)(milliseconds to wait=u32 1000 ("等待时间（毫秒）")) -> ()  [unwired: 1 out]
                  }
                  frame #1 {
                    w1000 = u16 256 ("y")
                    w1015 = u8 0 ("元素")
                    n578 = local read "目标板类型"() -> (w990:enum16{"BCU/主板", "BMU/从板"})
                    n579 = case shown="\"BCU/主板\", 默认" w990 {
                      tunnel: [u16 0 ("请选择板号") w1022] -> w989
                      frame "BCU/主板", Default {
                      }
                      frame "BMU/从板" {
                        n580 = local read "请选择板号"() -> (w1022:u16)
                      }
                    }
                    n581 = local read "设备索引"() -> (w1010:u32)
                    n582 = local read "CAN路数"() -> (w1009:u32)
                    n583 = local read "类型"() -> (w1011:u32)
                    n584 = Multiply(x=w989, y=w1000) -> ()  [unwired: 1 out]
                    n585 = Multiply(x=w1000, y=w999) -> (x*y=w998:u16)
                    n586 = local read "Info："() -> (w1004:string)
                    n587 = Add(x=u32 131217 ("ID"), y=w998) -> (x+y=w1005:u32)
                    n588 = local read "VCI_CAN_OBJ_T"() -> (w1008:T1)
                    n589 = local read "CRC16"() -> (w997:u16)
                    n590 = Concatenate Strings(w1004, "boot就绪查询..." ("字符串"), "\n") -> (w1001:string)
                    n591 = Split Number(x=w997) -> (hi(x)=w995:u8, lo(x)=w996:u8)
                    n592 = local write "Info："(w1001) -> ()
                    n593 = Bundle(cluster=w1008, "ID"=w1005, "TimeStamp"=u8 0 ("RemoteFlag"), "TimeFlag"=u8 1, "SendType"=u8 0 ("DataLen"), "RemoteFlag"=u8 0, "ExternFlag"=u8 1, "DataLen"=u8 8, u8 1 ("元素"), w994, w993, w992, w991, w995, w996, w1015, w1015, w1015) -> (w1012:T1)  [unwired: 1 in]
                    n594 = dll-call lib="F:/Bluewave New Energy/SVN_Work/AutoTest_TestStand/trunk/AutoTest_TestStand/Driver/ZlgCan/BHN01/AutoBurn/Settings/ControlCAN.dll" fn="VCI_Transmit"("DeviceType"=w1011, "DeviceInd"=w1010, "CANInd"=w1009, "pSend"=w1012, "Len"=u32 1) -> ()  [unwired: 5 in, 6 out]
                  }
                }
                n595 = local read "Info："() -> (w979:string)
                n596 = local write "进入烧录"(FALSE ("进入烧录")) -> ()
                n597 = Concatenate Strings(w979, "boot模式应答...成功" ("字符串"), "\n") -> (w982:string)
                n598 = local write "Info："(w982) -> ()
                "boot模式应答...成功" <- TRUE
              }
            }
          }
          frame 168192..168224, 168447 {
            n599 = To Unsigned Byte Integer(number=w1025) -> (unsigned 8bit integer=w1024:u8)
            n600 = Equal?(x=w1027, y=u8 85) -> (x = y?=w1023:bool)
            n601 = case shown="假" w1023 {
              tunnel: w1024 -> [_ w1048]
              frame False {
                n602 = disable-structure shown="禁用" {
                  frame Disabled {
                    n603 = flat-sequence {
                      frame #0 {
                        n604 = local read "设备索引"() -> (w1041:u32)
                        n605 = local read "CAN路数"() -> (w1039:u32)
                        n606 = local read "波特率"() -> (w1040:T2)
                        n607 = local read "滤波方式"() -> (w1038:u8)
                        n608 = local read "工作方式"() -> (w1037:u8)
                        n609 = local read "类型"() -> (w1042:u32)
                        n610 = call "CAN_Init.vi"("设备类型"=w1042, "设备索引"=w1041, "波特率"=w1040, "CAN路数"=w1039, "操作类型"=enum16{"初始化CAN", "关闭CAN"}."关闭CAN", 6:w1038, 10:w1037) -> ()  [unwired: 12 in, 1 out]
                        n611 = Wait (ms)(milliseconds to wait=u32 2000 ("等待时间（毫秒）")) -> ()  [unwired: 1 out]
                      }
                      frame #1 {
                        n612 = Quit LabVIEW(quit? (T)=TRUE ("退出？(T)")) -> ()
                      }
                    }
                  }
                  frame Enabled {
                  }
                }
                n613 = local write "update flag"(FALSE ("update flag")) -> ()
                n614 = local read "Info："() -> (w1031:string)
                n615 = local write "退出？(T)"(TRUE ("退出？(T)")) -> ()
                n616 = Concatenate Strings(w1031, "boot就绪应答...失败" ("字符串"), "\n") -> (w1034:string)
                n617 = One Button Dialog(message="程序下载错误，请断电重试！" ("消息")) -> ()  [unwired: 1 in, 1 out]
                n618 = local write "Info："(w1034) -> ()
              }
              frame True {
                n619 = stacked-sequence {
                  tunnel: w1048 -> [_ w1057]
                  frame #0 {
                    n620 = disable-structure shown="启用" {
                      frame Enabled {
                        n621 = local read "CAN路数"() -> (w1051:u32)
                        n622 = local read "设备索引"() -> (w1052:u32)
                        n623 = local read "类型"() -> (w1053:u32)
                        n624 = dll-call lib="F:/Bluewave New Energy/SVN_Work/AutoTest_TestStand/trunk/AutoTest_TestStand/Driver/ZlgCan/BHN01/AutoBurn/Settings/ControlCAN.dll" fn="VCI_ClearBuffer" label="VCI_Clearbuffer"(error in=errorcluster {"status"=FALSE, "code"=0, "source"=""} ("错误输入（无错误）"), "DeviceType"=w1053, "DeviceInd"=w1052, "CANInd"=w1051) -> (error out=→"错误输出 13":errorcluster)  [unwired: 3 in, 4 out]
                      }
                      frame Disabled {
                      }
                    }
                  }
                  frame #1 {
                    w1058 = u16 256 ("y")
                    w1073 = u8 0 ("元素")
                    n625 = local read "目标板类型"() -> (w1055:enum16{"BCU/主板", "BMU/从板"})
                    n626 = case shown="\"BCU/主板\", 默认" w1055 {
                      tunnel: [u16 0 ("请选择板号") w1080] -> w1054
                      frame "BCU/主板", Default {
                      }
                      frame "BMU/从板" {
                        n627 = local read "请选择板号"() -> (w1080:u16)
                      }
                    }
                    n628 = local read "设备索引"() -> (w1068:u32)
                    n629 = local read "CAN路数"() -> (w1067:u32)
                    n630 = local read "类型"() -> (w1069:u32)
                    n631 = local read "Info："() -> (w1059:string)
                    n632 = Multiply(x=w1054, y=w1058) -> ()  [unwired: 1 out]
                    n633 = Multiply(x=w1058, y=w1057) -> (x*y=w1056:u16)
                    n634 = Concatenate Strings(w1059, "boot擦除flash请求..." ("字符串"), "\n") -> (w1062:string)
                    n635 = Add(x=u32 196753 ("ID"), y=w1056) -> (x+y=w1063:u32)
                    n636 = local write "Info："(w1062) -> ()
                    n637 = local read "VCI_CAN_OBJ_T"() -> (w1066:T1)
                    n638 = Bundle(cluster=w1066, "ID"=w1063, "TimeStamp"=u8 0 ("RemoteFlag"), "TimeFlag"=u8 1, "SendType"=u8 0 ("DataLen"), "RemoteFlag"=u8 0, "ExternFlag"=u8 1, "DataLen"=u8 8, u8 1 ("元素"), w1073, w1073, w1073) -> (w1070:T1)  [unwired: 7 in]
                    n639 = dll-call lib="F:/Bluewave New Energy/SVN_Work/AutoTest_TestStand/trunk/AutoTest_TestStand/Driver/ZlgCan/BHN01/AutoBurn/Settings/ControlCAN.dll" fn="VCI_Transmit"("DeviceType"=w1069, "DeviceInd"=w1068, "CANInd"=w1067, "pSend"=w1070, "Len"=u32 1) -> ()  [unwired: 5 in, 6 out]
                  }
                }
                n640 = local read "Info："() -> (w1044:string)
                n641 = Concatenate Strings(w1044, "boot就绪应答...成功" ("字符串"), "\n") -> (w1047:string)
                n642 = local write "Info："(w1047) -> ()
              }
            }
          }
          frame 233728..233760, 233983 {
            n643 = To Unsigned Byte Integer(number=w1082) -> (unsigned 8bit integer=w1081:u8)
            n644 = Equal?(x=w1089, y=u8 85) -> (x = y?=w1087:bool)
            n645 = case shown="假" w1087 {
              tunnel: w1086 -> [_ w1121]
              tunnel: w1085 -> [_ w1120]
              tunnel: w1084 -> [_ w1119]
              tunnel: w1083 -> [_ w1118]
              tunnel: w1081 -> [_ w1115]
              frame False {
                n646 = local write "update flag"(FALSE ("update flag")) -> ()
                n647 = local read "Info："() -> (w1093:string)
                n648 = Concatenate Strings(w1093, "boot擦除flash应答...失败" ("字符串"), "\n") -> (w1096:string)
                n649 = local write "Info："(w1096) -> ()
                n650 = One Button Dialog(message="程序下载错误，请断电重试！" ("消息")) -> ()  [unwired: 1 in, 1 out]
                n651 = disable-structure shown="禁用" {
                  frame Disabled {
                    n652 = flat-sequence {
                      frame #0 {
                        n653 = local read "设备索引"() -> (w1103:u32)
                        n654 = local read "CAN路数"() -> (w1101:u32)
                        n655 = local read "波特率"() -> (w1102:T2)
                        n656 = local read "滤波方式"() -> (w1100:u8)
                        n657 = local read "工作方式"() -> (w1099:u8)
                        n658 = local read "类型"() -> (w1104:u32)
                        n659 = call "CAN_Init.vi"("设备类型"=w1104, "设备索引"=w1103, "波特率"=w1102, "CAN路数"=w1101, "操作类型"=enum16{"初始化CAN", "关闭CAN"}."关闭CAN", 6:w1100, 10:w1099) -> ()  [unwired: 12 in, 1 out]
                        n660 = Wait (ms)(milliseconds to wait=u32 2000 ("等待时间（毫秒）")) -> ()  [unwired: 1 out]
                      }
                      frame #1 {
                        n661 = Quit LabVIEW(quit? (T)=TRUE ("退出？(T)")) -> ()
                      }
                    }
                  }
                  frame Enabled {
                  }
                }
                n662 = local write "退出？(T)"(TRUE ("退出？(T)")) -> ()
              }
              frame True {
                w1116 = 0 ("索引")
                n663 = local read "子数组"() -> (w1117:string[])
                n664 = flat-sequence {
                  frame #0 {
                    n665 = local read "Info："() -> (w1126:string)
                    n666 = Concatenate Strings(w1126, "boot擦除flash应答...成功" ("字符串"), "\n") -> (w1128:string)
                    n667 = local write "Info："(w1128) -> ()
                  }
                  frame #1 {
                    n668 = local read "Info："() -> (w1133:string)
                    n669 = Concatenate Strings(w1133, "开始下载数据..." ("字符串"), "\n") -> (w1131:string)
                    n670 = Tick Count (ms)() -> (millisecond timer value=w1129:u32)
                    n671 = local write "Info："(w1131) -> ()
                    n672 = local write "开始下载数据"(w1129) -> ()
                    "开始下载数据" <- TRUE
                  }
                }
                n673 = Array Size(array=w1117) -> (size(s)=w1122:i32)
                n674 = Index Array(array=w1117, index=w1116) -> (element=w1106:string)
                n675 = String Subset(string=w1106, offset (0)=1 ("偏移量(0)"), length (rest)=1 ("长度（子字符串长度）")) -> (substring=w1111:string)
                n676 = case shown="\"2\"" w1111 {
                  tunnel: ["01" ("子字符串(\"\")") "02" ("子字符串(\"\")")] -> w1110
                  frame "1", Default {
                  }
                  frame "2" {
                  }
                }
                n677 = String Subset(string=w1106, offset (0)=2 ("偏移量(0)")) -> (substring=w1108:string)  [unwired: 1 in]
                n678 = Concatenate Strings("FFFFFFFFFFFF" ("子字符串(\"\")"), w1110, w1108) -> ()  [unwired: 1 out]
                n679 = while {
                  tunnel: w1121 -> [w1158]
                  tunnel: w1120 -> [w1157]
                  tunnel: w1119 -> [w1156]
                  tunnel: w1118 -> [w1155]
                  shift-right: [w1150] -> _
                  shift-left: w1106 -> [w1151]
                  tunnel: w1122 -> [w1148]
                  tunnel: w1116 -> [w1144]
                  tunnel: w1115 -> [w1138]
                  tunnel: u16 1 ("y") -> [w1137]
                  stop <- w1143 stop-if-true
                  w1141 = u16 256 ("y")
                  n680 = String Length(string=w1151) -> (length=w1149:i32)
                  n681 = Greater Or Equal?(x=w1149, y=16) -> (x >= y?=w1152:bool)
                  n682 = local read "目标板类型"() -> (w1136:enum16{"BCU/主板", "BMU/从板"})
                  n683 = case shown="\"BCU/主板\", 默认" w1136 {
                    tunnel: [u16 0 ("请选择板号") w1160] -> w1135
                    frame "BCU/主板", Default {
                    }
                    frame "BMU/从板" {
                      n684 = local read "请选择板号"() -> (w1160:u16)
                    }
                  }
                  n685 = Multiply(x=w1135, y=w1141) -> ()  [unwired: 1 out]
                  n686 = Multiply(x=w1141, y=w1138) -> (x*y=w1140:u16)
                  n687 = Divide(x=w1144, y=w1148) -> (x/y=w1147:dbl)
                  n688 = Add(x=u32 262289 ("ID"), y=w1140) -> (x+y=w1139:u32)
                  n689 = Multiply(x=w1147, y=100.0) -> (x*y=w1145:dbl)
                  n690 = case shown="假" w1152 {
                    tunnel: w1158 -> [w1189 w1201]
                    tunnel: w1157 -> [w1188 w1200]
                    tunnel: w1156 -> [w1187 w1199]
                    tunnel: w1155 -> [w1186 w1198]
                    tunnel: w1151 -> [w1162 w1197]
                    tunnel: [w1167 w1196] -> w1150
                    tunnel: [FALSE TRUE] -> w1143
                    tunnel: w1149 -> [_ w1194]
                    tunnel: w1149 -> [_ w1193]
                    tunnel: w1139 -> [w1165 w1192]
                    tunnel: w1137 -> [_ w1191]
                    frame True {
                      w1183 = u8 0 ("元素")
                      n691 = String Subset(string=w1162, length (rest)=16 ("长度（剩余）")) -> (substring=w1161:string)  [unwired: 1 in]
                      n692 = String Subset(string=w1162, offset (0)=16 ("偏移量(0)")) -> (substring=w1167:string)  [unwired: 1 in]
                      n693 = call "ASCII_To_Hex.vi"("ASCII String"=w1161) -> ("hex数组"=w1163:u16[])  [unwired: 6 in, 4 out]
                      n694 = Index Array(array=w1163) -> (element #1=w1175:u16, element #2=w1174:u16, element #3=w1173:u16, element #4=w1172:u16, element #5=w1171:u16, element #6=w1170:u16, element #7=w1169:u16, element #8=w1168:u16)  [unwired: 8 in]
                      n695 = Bundle(cluster=w1189, "ID"=w1165, "TimeStamp"=u8 0 ("RemoteFlag"), "TimeFlag"=u8 1, "SendType"=u8 0 ("DataLen"), "RemoteFlag"=u8 0, "ExternFlag"=u8 1, "DataLen"=u8 8, w1175, w1174, w1173, w1172, w1171, w1170, w1169, w1168, w1183, w1183, w1183) -> (w1178:T1)
                      n696 = dll-call lib="F:/Bluewave New Energy/SVN_Work/AutoTest_TestStand/trunk/AutoTest_TestStand/Driver/ZlgCan/BHN01/AutoBurn/Settings/ControlCAN.dll" fn="VCI_Transmit"("DeviceType"=w1188, "DeviceInd"=w1187, "CANInd"=w1186, "pSend"=w1178, "Len"=u32 1) -> ()  [unwired: 5 in, 6 out]
                    }
                    frame False {
                      n697 = Greater Than 0?(x=w1194) -> (x > 0?=w1190:bool)
                      n698 = case shown="真" w1190 {
                        tunnel: w1201 -> [w1232 w1242]
                        tunnel: w1200 -> [w1231 w1241]
                        tunnel: w1199 -> [w1230 w1240]
                        tunnel: w1198 -> [w1229 w1239]
                        tunnel: w1197 -> [w1219 _]
                        tunnel: [w1210 _] -> w1196
                        tunnel: w1193 -> [_ w1237]
                        tunnel: w1192 -> [w1206 w1236]
                        tunnel: w1191 -> [_ w1235]
                        tunnel: w1191 -> [w1205 _]
                        frame True {
                          w1226 = u8 0 ("元素")
                          n699 = Wait (ms)(milliseconds to wait=u32 20 ("等待时间（毫秒）")) -> ()  [unwired: 1 out]
                          n700 = String Subset(string=w1219, offset (0)=16 ("偏移量(0)")) -> (substring=w1210:string)  [unwired: 1 in]
                          n701 = String Subset(string=w1219, length (rest)=16 ("长度（剩余）")) -> (substring=w1203:string)  [unwired: 1 in]
                          n702 = call "ASCII_To_Hex.vi"("ASCII String"=w1203) -> ("hex数组"=w1202:u16[])  [unwired: 6 in, 4 out]
                          n703 = Index Array(array=w1202) -> (element #1=w1218:u16, element #2=w1217:u16, element #3=w1216:u16, element #4=w1215:u16, element #5=w1214:u16, element #6=w1213:u16, element #7=w1212:u16, element #8=w1211:u16)  [unwired: 8 in]
                          n704 = Bundle(cluster=w1232, "ID"=w1206, "TimeStamp"=u8 0 ("RemoteFlag"), "TimeFlag"=u8 1, "SendType"=u8 0 ("DataLen"), "RemoteFlag"=u8 0, "ExternFlag"=w1205, "DataLen"=u8 8, w1218, w1217, w1216, w1215, w1214, w1213, w1212, w1211, w1226, w1226, w1226) -> (w1221:T1)
                          n705 = dll-call lib="F:/Bluewave New Energy/SVN_Work/AutoTest_TestStand/trunk/AutoTest_TestStand/Driver/ZlgCan/BHN01/AutoBurn/Settings/ControlCAN.dll" fn="VCI_Transmit"(error in="错误输入（无错误） 3", "DeviceType"=w1231, "DeviceInd"=w1230, "CANInd"=w1229, "pSend"=w1221, "Len"=u32 1) -> (error out=→"错误输出 14":errorcluster)  [unwired: 4 in, 5 out]
                        }
                        frame False {
                          (unwired) TRUE
                          n706 = Quotient & Remainder(x=w1237, y=8) -> ()  [unwired: 2 out]
                          n707 = Wait (ms)(milliseconds to wait=u32 20 ("等待时间（毫秒）")) -> ()  [unwired: 1 out]
                          n708 = case shown="0" 1 {
                            tunnel: w1242 -> [w1267 _]
                            tunnel: w1241 -> [w1266 _]
                            tunnel: w1240 -> [w1265 _]
                            tunnel: w1239 -> [w1264 _]
                            tunnel: w1236 -> [w1244 _]
                            tunnel: w1235 -> [w1243 _]
                            frame 0 {
                              w1261 = u8 0 ("元素")
                              n709 = Index Array(array=u8[] [0, 0, 0, 0, 0, 0, 0, 0] ("数组")) -> (element #1=w1255:u8, element #2=w1254:u8, element #3=w1253:u8, element #4=w1252:u8, element #5=w1251:u8, element #6=w1250:u8, element #7=w1249:u8, element #8=w1248:u8)  [unwired: 8 in]
                              n710 = Bundle(cluster=w1267, "ID"=w1244, "TimeStamp"=u8 0 ("RemoteFlag"), "TimeFlag"=u8 1, "SendType"=u8 0 ("DataLen"), "RemoteFlag"=u8 0, "ExternFlag"=w1243, "DataLen"=u8 8, w1255, w1254, w1253, w1252, w1251, w1250, w1249, w1248, w1261, w1261, w1261) -> (w1256:T1)
                              n711 = dll-call lib="F:/Bluewave New Energy/SVN_Work/AutoTest_TestStand/trunk/AutoTest_TestStand/Driver/ZlgCan/BHN01/AutoBurn/Settings/ControlCAN.dll" fn="VCI_Transmit"(error in="错误输入（无错误） 4", "DeviceType"=w1266, "DeviceInd"=w1265, "CANInd"=w1264, "pSend"=w1256, "Len"=u32 1) -> (error out=→"错误输出 15":errorcluster)  [unwired: 4 in, 5 out]
                            }
                            frame 1, Default {
                            }
                          }
                        }
                      }
                    }
                  }
                  n712 = local write "进度"(w1145) -> ()
                  n713 = Wait (ms)(milliseconds to wait=u32 5 ("等待时间（毫秒）")) -> ()  [unwired: 1 out]
                }
                "当前发送行" <- w1116
              }
            }
          }
          frame 299264..299296, 299519 {
            n714 = To Unsigned Byte Integer(number=w1271) -> (unsigned 8bit integer=w1270:u8)
            n715 = Equal?(x=w1269, y=u8 85) -> (x = y?=w1268:bool)
            n716 = case shown="真" w1268 {
              tunnel: w1275 -> [_ w1301]
              tunnel: w1274 -> [_ w1300]
              tunnel: w1273 -> [_ w1299]
              tunnel: w1272 -> [_ w1298]
              tunnel: w1270 -> [_ w1292]
              frame False {
                n717 = local write "update flag"(FALSE ("update flag")) -> ()
                n718 = local read "Info："() -> (w1279:string)
                n719 = Concatenate Strings(w1279, "扇区数据传输应答...失败" ("字符串"), "\n") -> (w1282:string)
                n720 = One Button Dialog(message="程序下载错误，请断电重试！" ("消息")) -> ()  [unwired: 1 in, 1 out]
                n721 = local write "Info："(w1282) -> ()
              }
              frame True {
                n722 = local read "当前发送行"() -> (w1296:i32)
                n723 = local read "子数组"() -> (w1297:string[])
                n724 = Array Size(array=w1297) -> (size(s)=w1302:i32)
                n725 = Increment(x=w1296) -> (x+1=w1295:i32)
                n726 = Index Array(array=w1297, index=w1295) -> (element=w1284:string)
                n727 = String Subset(string=w1284, offset (0)=1 ("偏移量(0)"), length (rest)=1 ("长度（子字符串长度）")) -> (substring=w1289:string)
                n728 = case shown="\"2\"" w1289 {
                  tunnel: ["01" ("子字符串(\"\")") "02" ("子字符串(\"\")")] -> w1287
                  frame "1", Default {
                  }
                  frame "2" {
                  }
                }
                n729 = Tick Count (ms)() -> (millisecond timer value=w1283:u32)
                n730 = local write "当前发送行"(w1295) -> ()
                n731 = String Subset(string=w1284, offset (0)=2 ("偏移量(0)")) -> (substring=w1285:string)  [unwired: 1 in]
                n732 = String Length(string=w1284) -> (length=w1294:i32)
                n733 = local write "开始下载数据"(w1283) -> ()
                n734 = Concatenate Strings("FFFFFFFFFFFF" ("子字符串(\"\")"), w1287, w1285) -> ()  [unwired: 1 out]
                n735 = Greater Than 0?(x=w1294) -> (x > 0?=w1293:bool)
                n736 = case shown="假" w1293 {
                  tunnel: w1302 -> [_ w1359]
                  tunnel: w1301 -> [w1347 w1358]
                  tunnel: w1300 -> [w1346 w1357]
                  tunnel: w1299 -> [w1345 w1356]
                  tunnel: w1298 -> [w1344 w1355]
                  tunnel: w1295 -> [_ w1354]
                  tunnel: w1284 -> [_ w1353]
                  tunnel: w1292 -> [w1317 w1348]
                  frame False {
                    w1308 = "BURNRESULT" ("section")
                    w1341 = u8 0 ("元素")
                    n737 = Multiply(x=w1317, y=u16 256) -> (x*y=w1314:u16)
                    n738 = local write "update flag"(FALSE ("update flag")) -> ()
                    n739 = local write "开始下载数据"(FALSE ("开始下载数据")) -> ()
                    n740 = Add(x=u32 327825 ("ID"), y=w1314) -> (x+y=w1315:u32)
                    n741 = String To Byte Array(string="" ("字符串")) -> (unsigned byte array=w1335:u8[])
                    n742 = Index Array(array=w1335) -> (element #1=w1334:u8, element #2=w1333:u8, element #3=w1332:u8, element #4=w1331:u8, element #5=w1330:u8, element #6=w1329:u8, element #7=w1328:u8, element #8=w1327:u8)  [unwired: 8 in]
                    n743 = local read "Info："() -> (w1320:string)
                    n744 = Concatenate Strings(w1320, "应用刷写完成..请重新上电！" ("字符串"), "\n") -> (w1323:string)
                    n745 = local write "Info："(w1323) -> ()
                    n746 = call <vilib>:"Open Config Data.vi"("configuration file path"=path "D:/BlueWay/configresult.ini") -> ("refnum"=w1307:T4)  [unwired: 8 in, 2 out]
                    n747 = Bundle(cluster=w1347, "ID"=w1315, "TimeStamp"=u8 0 ("RemoteFlag"), "TimeFlag"=u8 1, "SendType"=u8 0 ("DataLen"), "RemoteFlag"=u8 0, "ExternFlag"=u8 1, "DataLen"=u8 8, w1334, w1333, w1332, w1331, w1330, w1329, w1328, w1327, w1341, w1341, w1341) -> (w1336:T1)
                    n748 = call-poly <vilib>:"Write Key.vi"("section"=w1308, "value"="PASS" ("section"), "key"=w1308, "refnum"=w1307) -> ("error out"=w1311:errorcluster, "refnum out"=w1310:T4)  [unwired: 5 in, 1 out]
                    n749 = dll-call lib="F:/Bluewave New Energy/SVN_Work/AutoTest_TestStand/trunk/AutoTest_TestStand/Driver/ZlgCan/BHN01/AutoBurn/Settings/ControlCAN.dll" fn="VCI_Transmit"(error in="错误输入（无错误） 7", "DeviceType"=w1346, "DeviceInd"=w1345, "CANInd"=w1344, "pSend"=w1336, "Len"=u32 1) -> (error out=→"错误输出 18":errorcluster)  [unwired: 4 in, 5 out]
                    n750 = call <vilib>:"Close Config Data.vi"("error in (no error)"=w1311, "refnum"=w1310) -> ()  [unwired: 8 in, 2 out]
                    n751 = local write "退出？(T)"(TRUE ("退出？(T)")) -> ()
                  }
                  frame True {
                    n752 = Multiply(x=w1348, y=u16 256) -> (x*y=w1351:u16)
                    n753 = Add(x=u32 262289 ("ID"), y=w1351) -> (x+y=w1349:u32)
                    n754 = while {
                      tunnel: w1358 -> [w1375]
                      tunnel: w1357 -> [w1374]
                      tunnel: w1356 -> [w1373]
                      tunnel: w1355 -> [w1372]
                      shift-right: [w1368] -> _
                      shift-left: w1353 -> [w1369]
                      tunnel: w1359 -> [w1366]
                      tunnel: w1354 -> [w1362]
                      tunnel: w1349 -> [w1360]
                      stop <- w1361 stop-if-true
                      n755 = String Length(string=w1369) -> (length=w1367:i32)
                      n756 = Greater Or Equal?(x=w1367, y=16) -> (x >= y?=w1370:bool)
                      n757 = case shown="真" w1370 {
                        tunnel: w1375 -> [w1404 w1416]
                        tunnel: w1374 -> [w1403 w1415]
                        tunnel: w1373 -> [w1402 w1414]
                        tunnel: w1372 -> [w1401 w1413]
                        tunnel: w1369 -> [w1391 w1412]
                        tunnel: [w1381 w1411] -> w1368
                        tunnel: [FALSE TRUE] -> w1361
                        tunnel: w1367 -> [_ w1409]
                        tunnel: w1367 -> [_ w1408]
                        tunnel: w1360 -> [w1379 w1406]
                        frame True {
                          (unwired) u8 1 ("ExternFlag")
                          w1398 = u8 0 ("元素")
                          n758 = String Subset(string=w1391, offset (0)=16 ("偏移量(0)")) -> (substring=w1381:string)  [unwired: 1 in]
                          n759 = String Subset(string=w1391, length (rest)=16 ("长度（剩余）")) -> (substring=w1377:string)  [unwired: 1 in]
                          n760 = call "ASCII_To_Hex.vi"("ASCII String"=w1377) -> ("hex数组"=w1376:u16[])  [unwired: 6 in, 4 out]
                          n761 = Index Array(array=w1376) -> (element #1=w1389:u16, element #2=w1388:u16, element #3=w1387:u16, element #4=w1386:u16, element #5=w1385:u16, element #6=w1384:u16, element #7=w1383:u16, element #8=w1382:u16)  [unwired: 8 in]
                          n762 = Bundle(cluster=w1404, "ID"=w1379, "TimeStamp"=u8 0 ("RemoteFlag"), "TimeFlag"=u8 1, "SendType"=u8 0 ("DataLen"), "RemoteFlag"=u8 0, "ExternFlag"=u8 1, "DataLen"=u8 8, w1389, w1388, w1387, w1386, w1385, w1384, w1383, w1382, w1398, w1398, w1398) -> (w1393:T1)
                          n763 = dll-call lib="F:/Bluewave New Energy/SVN_Work/AutoTest_TestStand/trunk/AutoTest_TestStand/Driver/ZlgCan/BHN01/AutoBurn/Settings/ControlCAN.dll" fn="VCI_Transmit"("DeviceType"=w1403, "DeviceInd"=w1402, "CANInd"=w1401, "pSend"=w1393, "Len"=u32 1) -> ()  [unwired: 5 in, 6 out]
                        }
                        frame False {
                          n764 = Greater Than 0?(x=w1409) -> ()  [unwired: 1 out]
                          n765 = case shown="真" TRUE {
                            tunnel: w1416 -> [w1447 w1454]
                            tunnel: w1415 -> [w1446 w1453]
                            tunnel: w1414 -> [w1445 w1452]
                            tunnel: w1413 -> [w1444 w1451]
                            tunnel: w1412 -> [w1434 _]
                            tunnel: [w1425 _] -> w1411
                            tunnel: w1408 -> [_ w1449]
                            tunnel: w1406 -> [w1422 _]
                            tunnel: [w1420 _] -> w1405
                            frame True {
                              w1441 = u8 0 ("元素")
                              n766 = String Subset(string=w1434, length (rest)=16 ("长度（剩余）")) -> (substring=w1419:string)  [unwired: 1 in]
                              n767 = String Subset(string=w1434, offset (0)=16 ("偏移量(0)")) -> (substring=w1425:string)  [unwired: 1 in]
                              n768 = call "ASCII_To_Hex.vi"("ASCII String"=w1419) -> ("hex数组"=w1418:u16[])  [unwired: 6 in, 4 out]
                              n769 = Index Array(array=w1418) -> (element #1=w1433:u16, element #2=w1432:u16, element #3=w1431:u16, element #4=w1430:u16, element #5=w1429:u16, element #6=w1428:u16, element #7=w1427:u16, element #8=w1426:u16)  [unwired: 8 in]
                              n770 = Bundle(cluster=w1447, "ID"=w1422, "TimeStamp"=u8 0 ("RemoteFlag"), "TimeFlag"=u8 1, "SendType"=u8 0 ("DataLen"), "RemoteFlag"=u8 0, "ExternFlag"=u8 1, "DataLen"=u8 8, w1433, w1432, w1431, w1430, w1429, w1428, w1427, w1426, w1441, w1441, w1441) -> (w1436:T1)
                              n771 = dll-call lib="F:/Bluewave New Energy/SVN_Work/AutoTest_TestStand/trunk/AutoTest_TestStand/Driver/ZlgCan/BHN01/AutoBurn/Settings/ControlCAN.dll" fn="VCI_Transmit"(error in="错误输入（无错误） 5", "DeviceType"=w1446, "DeviceInd"=w1445, "CANInd"=w1444, "pSend"=w1436, "Len"=u32 1) -> (error out=w1420:errorcluster)  [unwired: 4 in, 5 out]
                              "错误输出 16" <- w1420
                            }
                            frame False {
                              n772 = Quotient & Remainder(x=w1449, y=8) -> (x-y*floor(x/y)=w1448:i32)  [unwired: 1 out]
                              n773 = case shown="0" w1448 {
                                tunnel: w1454 -> [w1478 _]
                                tunnel: w1453 -> [w1477 _]
                                tunnel: w1452 -> [w1476 _]
                                tunnel: w1451 -> [w1475 _]
                                frame 0 {
                                w1471 = u8 0 ("元素")
                                n774 = Index Array(array=u8[] [0, 0, 0, 0, 0, 0, 0, 0] ("数组")) -> (element #1=w1465:u8, element #2=w1464:u8, element #3=w1463:u8, element #4=w1462:u8, element #5=w1461:u8, element #6=w1460:u8, element #7=w1459:u8, element #8=w1458:u8)  [unwired: 8 in]
                                n775 = Bundle(cluster=w1478, "ID"=u32 5, "TimeStamp"=u8 0 ("RemoteFlag"), "TimeFlag"=u8 1, "SendType"=u8 0 ("DataLen"), "RemoteFlag"=u8 0, "DataLen"=u8 8, w1465, w1464, w1463, w1462, w1461, w1460, w1459, w1458, w1471, w1471, w1471) -> (w1466:T1)  [unwired: 1 in]
                                n776 = dll-call lib="F:/Bluewave New Energy/SVN_Work/AutoTest_TestStand/trunk/AutoTest_TestStand/Driver/ZlgCan/BHN01/AutoBurn/Settings/ControlCAN.dll" fn="VCI_Transmit"(error in="错误输入（无错误） 6", "DeviceType"=w1477, "DeviceInd"=w1476, "CANInd"=w1475, "pSend"=w1466, "Len"=u32 1) -> (error out=→"错误输出 17":errorcluster)  [unwired: 4 in, 5 out]
                                }
                                frame 1, Default {
                                }
                              }
                            }
                          }
                          n777 = flat-sequence {
                            tunnel: w1405 -> [_]
                            frame #0 {
                              n778 = Wait (ms)(milliseconds to wait=u32 1 ("等待时间（毫秒）")) -> ()  [unwired: 1 out]
                            }
                          }
                        }
                      }
                      n779 = Divide(x=w1362, y=w1366) -> (x/y=w1365:dbl)
                      n780 = Multiply(x=w1365, y=100.0) -> (x*y=w1363:dbl)
                      n781 = local write "进度"(w1363) -> ()
                    }
                  }
                }
              }
            }
          }
          frame 254 {
            (unwired) TRUE
            n782 = disable-structure shown="禁用" {
              disable-tunnel: w1485 -> [w1495 _]
              disable-tunnel: w1484 -> [w1494 _]
              disable-tunnel: w1483 -> [w1493 _]
              disable-tunnel: w1482 -> [w1492 _]
              disable-tunnel: w1479 -> [w1488 _]
              frame Disabled {
                w1491 = FALSE ("进入烧录模式")
                n783 = Two Button Dialog(message="进入烧录模式!，是否开始烧录？\n如果BMS重新上电，请点取消！！" ("消息")) -> (T button?=w1486:bool)  [unwired: 2 in]
                n784 = case shown="真" w1486 {
                  tunnel: w1495 -> [w1501 w1528]
                  tunnel: w1494 -> [w1500 w1523]
                  tunnel: w1493 -> [w1499 w1522]
                  tunnel: w1492 -> [w1498 w1521]
                  tunnel: w1488 -> [w1496 w1524]
                  frame True {
                    n785 = stacked-sequence {
                      tunnel: w1501 -> [_ w1509]
                      tunnel: w1500 -> [w1504 w1508]
                      tunnel: w1499 -> [w1503 w1507]
                      tunnel: w1498 -> [w1502 w1506]
                      tunnel: w1496 -> [w1505 _]
                      frame #0 {
                        n786 = Flush Queue(queue=w1505) -> ()  [unwired: 1 in, 3 out]
                        n787 = dll-call lib="F:/Bluewave New Energy/SVN_Work/AutoTest_TestStand/trunk/AutoTest_TestStand/Driver/ZlgCan/BHN01/AutoBurn/Settings/ControlCAN.dll" fn="VCI_ClearBuffer" label="VCI_Clearbuffer"("DeviceType"=w1504, "DeviceInd"=w1503, "CANInd"=w1502) -> ()  [unwired: 4 in, 5 out]
                      }
                      frame #1 {
                        w1516 = u8 0 ("元素")
                        n788 = Bundle(cluster=w1509, "ID"=u32 0, "TimeStamp"=u8 0 ("RemoteFlag"), "TimeFlag"=u8 1, "SendType"=u8 0 ("DataLen"), "RemoteFlag"=u8 0, "ExternFlag"=u8 0, "DataLen"=u8 1, u8 2 ("元素"), w1516, w1516, w1516) -> (w1520:T1)  [unwired: 7 in]
                        n789 = dll-call lib="F:/Bluewave New Energy/SVN_Work/AutoTest_TestStand/trunk/AutoTest_TestStand/Driver/ZlgCan/BHN01/AutoBurn/Settings/ControlCAN.dll" fn="VCI_Transmit"("DeviceType"=w1508, "DeviceInd"=w1507, "CANInd"=w1506, "pSend"=w1520, "Len"=u32 1) -> ()  [unwired: 5 in, 6 out]
                      }
                    }
                    "进入烧录模式" <- TRUE ("进入烧录模式")
                  }
                  frame False {
                    n790 = Flush Queue(queue=w1524) -> (error out=w1526:errorcluster)  [unwired: 1 in, 2 out]
                    n791 = invoke on="Monitor" class="Bool" method="Reinit To Default"() -> ()  [unwired: 3 in, 3 out]
                    n792 = local write "Monitor_flag"(FALSE ("Monitor_flag")) -> ()
                    n793 = dll-call lib="F:/Bluewave New Energy/SVN_Work/AutoTest_TestStand/trunk/AutoTest_TestStand/Driver/ZlgCan/BHN01/AutoBurn/Settings/ControlCAN.dll" fn="VCI_ClearBuffer" label="VCI_Clearbuffer"(error in=w1526, "DeviceType"=w1523, "DeviceInd"=w1522, "CANInd"=w1521) -> (error out=w1525:errorcluster)  [unwired: 3 in, 4 out]
                    n794 = disable-structure shown="禁用" {
                      disable-tunnel: w1528 -> [w1533 _]
                      disable-tunnel: w1525 -> [w1532 _]
                      disable-tunnel: w1523 -> [w1531 _]
                      disable-tunnel: w1522 -> [w1530 _]
                      disable-tunnel: w1521 -> [w1529 _]
                      frame Disabled {
                        w1540 = u8 0 ("元素")
                        n795 = Bundle(cluster=w1533, "ID"=u32 0, "TimeStamp"=u8 0 ("RemoteFlag"), "TimeFlag"=u8 1, "SendType"=u8 0 ("DataLen"), "RemoteFlag"=u8 0, "ExternFlag"=u8 0, "DataLen"=u8 1, u8 5 ("元素"), w1540, w1540, w1540) -> (w1544:T1)  [unwired: 7 in]
                        n796 = dll-call lib="F:/Bluewave New Energy/SVN_Work/AutoTest_TestStand/trunk/AutoTest_TestStand/Driver/ZlgCan/BHN01/AutoBurn/Settings/ControlCAN.dll" fn="VCI_Transmit"(error in=w1532, "DeviceType"=w1531, "DeviceInd"=w1530, "CANInd"=w1529, "pSend"=w1544, "Len"=u32 1) -> ()  [unwired: 4 in, 6 out]
                      }
                      frame Enabled {
                      }
                    }
                  }
                }
                n797 = property on="烧录结果" class="Bool (严格)"("Colors [4]"=cluster{u32, u32}[] [{0, 0}] ("颜色[4]"), "BoolText.Text"="" ("布尔文本.文本")) -> ()  [unwired: 2 in, 2 out]
                n798 = local write "擦除完成"(w1491) -> ()
                n799 = local write "烧录结果"(w1491) -> ()
              }
              frame Enabled {
              }
            }
          }
          frame 253 {
            n800 = disable-structure shown="禁用" {
              disable-tunnel: w1554 -> [w1564 _]
              disable-tunnel: [w1563 _] -> w1553
              disable-tunnel: w1552 -> [w1562 _]
              disable-tunnel: w1551 -> [w1561 _]
              disable-tunnel: w1550 -> [w1560 _]
              disable-tunnel: w1549 -> [w1559 _]
              disable-tunnel: w1548 -> [w1558 _]
              disable-tunnel: [w1557 _] -> w1547
              disable-tunnel: w1546 -> [w1556 _]
              disable-tunnel: w1545 -> [w1555 _]
              frame Disabled {
                n801 = stacked-sequence {
                  tunnel: w1564 -> [_ w1582]
                  tunnel: [_ w1581] -> w1563
                  tunnel: w1562 -> [w1569 w1580]
                  tunnel: w1561 -> [w1568 w1579]
                  tunnel: w1560 -> [_ w1578]
                  tunnel: w1559 -> [w1567 w1577]
                  tunnel: w1558 -> [_ w1576]
                  tunnel: [_ w1575] -> w1557
                  tunnel: w1556 -> [_ w1574]
                  tunnel: w1555 -> [w1566 w1570]
                  frame #0 {
                    n802 = dll-call lib="F:/Bluewave New Energy/SVN_Work/AutoTest_TestStand/trunk/AutoTest_TestStand/Driver/ZlgCan/BHN01/AutoBurn/Settings/ControlCAN.dll" fn="VCI_ClearBuffer" label="VCI_Clearbuffer"("DeviceType"=w1569, "DeviceInd"=w1568, "CANInd"=w1567) -> ()  [unwired: 4 in, 5 out]
                    n803 = Flush Queue(queue=w1566) -> ()  [unwired: 1 in, 3 out]
                  }
                  frame #1 {
                    # "FD"
                    n804 = local read "子数组"() -> (w1584:string[])
                    n805 = while {
                      tunnel: w1584 -> [w1655] mode=indexing
                      tunnel: [w1651] -> w1583
                      tunnel: [w1647] -> w1573
                      i -> [w1651]
                      stop <- w1648 stop-if-true
                      n806 = Search/Split String(string=w1655, search string/char (-)="S9" ("搜索字符串/字符(-)")) -> (offset of match=w1653:i32)  [unwired: 1 in, 2 out]
                      n807 = Equal?(x=5000, y=w1651) -> (x = y?=w1649:bool)
                      n808 = Not Equal?(x=w1653, y=-1) -> (x != y?=w1647:bool)
                      n809 = Or(x=w1647, y=w1649) -> (x .or. y?=w1648:bool)
                    }
                    n810 = while {
                      tunnel: w1584 -> [w1664] mode=indexing
                      tunnel: [w1657] -> w1571
                      tunnel: [w1656] -> w1572
                      i -> [w1657]
                      stop <- w1659 stop-if-true
                      n811 = Equal?(x=5000, y=w1657) -> (x = y?=w1658:bool)
                      n812 = Search/Split String(string=w1664, search string/char (-)="S0" ("搜索字符串/字符(-)")) -> (offset of match=w1662:i32)  [unwired: 1 in, 2 out]
                      n813 = Not Equal?(x=w1662, y=-1) -> (x != y?=w1656:bool)
                      n814 = Or(x=w1656, y=w1658) -> (x .or. y?=w1659:bool)
                    }
                    n815 = case shown="真" w1573 {
                      tunnel: w1584 -> [_ w1630]
                      tunnel: w1583 -> [_ w1629]
                      tunnel: w1582 -> [w1586 _]
                      tunnel: [w1586 w1596] -> w1581
                      tunnel: w1580 -> [_ w1628]
                      tunnel: w1579 -> [_ w1627]
                      tunnel: w1578 -> [_ _]
                      tunnel: w1577 -> [_ w1626]
                      tunnel: w1576 -> [w1585 w1611]
                      tunnel: [w1585 w1609] -> w1575
                      tunnel: w1574 -> [_ w1593]
                      tunnel: w1572 -> [_ w1592]
                      tunnel: w1571 -> [_ w1591]
                      tunnel: w1570 -> [_ w1587]
                      frame False {
                      }
                      frame True {
                        n816 = case shown="真" w1592 {
                          tunnel: w1591 -> [_ w1633]
                          tunnel: [0 w1634] -> w1590
                          tunnel: [-1 w1633] -> w1589
                          frame False {
                          }
                          frame True {
                            n817 = Increment(x=w1633) -> (x+1=w1634:i32)
                          }
                        }
                        n818 = Subtract(x=w1629, y=w1589) -> (x-y=w1603:i32)
                        n819 = Decrement(x=w1603) -> (x-1=w1602:i32)
                        n820 = Array Subset(array=w1630, index=w1590, length=w1602) -> (w1600:string[])
                        n821 = Index Array(array=w1600, index=0 ("索引")) -> (element=w1608:string)
                        n822 = Delete From Array(array=w1600, length=1 ("长度"), index=0 ("索引")) -> (array with subset deleted=w1596:string[])  [unwired: 1 out]
                        n823 = String Subset(string=w1608, offset (0)=0 ("偏移量(0)"), length (rest)=2 ("长度（剩余）")) -> (substring=w1618:string)
                        n824 = String Subset(string=w1608, offset (0)=2 ("偏移量(0)"), length (rest)=2 ("长度（剩余）")) -> (substring=w1621:string)
                        n825 = Hexadecimal String To Number(string=w1621) -> (number=w1616:u32)  [unwired: 2 in, 1 out]
                        n826 = case shown="\"S2\"" w1618 {
                          tunnel: [4 ("偏移量(0)") 6 ("偏移量(0)")] -> w1607
                          tunnel: w1616 -> [w1639 w1645]
                          tunnel: [w1637 w1643] -> w1615
                          tunnel: [8 ("y") 10 ("y")] -> w1612
                          tunnel: ["S1" "S2"] -> w1604
                          frame "S1", Default {
                            n827 = Subtract(x=w1639, y=3) -> (x-y=w1637:u32)
                          }
                          frame "S2" {
                            n828 = Subtract(x=w1645, y=4) -> (x-y=w1643:u32)
                          }
                        }
                        "地址长度" <- w1607
                        n829 = Array Size(array=w1596) -> (size(s)=w1597:i32)
                        "大小" <- w1597
                        n830 = Divide(x=0, y=w1597) -> (x/y=w1594:dbl)
                        n831 = local write "进度"(w1594) -> ()
                        n832 = String Subset(string=w1608, offset (0)=4 ("偏移量(0)"), length (rest)=w1607) -> ()  [unwired: 1 out]
                        n833 = Multiply(x=u32 2, y=w1615) -> (x*y=w1613:u32)
                        "数据长度" <- w1613
                        n834 = String Subset(string=w1608, offset (0)=4 ("偏移量(0)"), length (rest)=w1607) -> (substring=w1605:string)
                        n835 = call "CAN R&W.vi"("设备类型"=w1628, "设备索引"=w1627, "CAN路数"=w1626, "DataLen"=u8 8, "写地址/数据"=enum16{"写地址", "写数据"}."写地址", "Data Input"=w1605, "枚举"=w1593, "TYPE"=w1604, "queue out"=w1587) -> ("发送的数据"=→"发送的数据":i32[])  [unwired: 17 in, 1 out]
                        n836 = String Subset(string=w1608, offset (0)=w1612, length (rest)=w1613) -> (substring=w1610:string)
                        n837 = Concatenate Strings(w1611, w1610) -> (w1609:string)
                      }
                    }
                  }
                }
                "擦除完成" <- TRUE ("擦写状态")
              }
              frame Enabled {
              }
            }
          }
          frame 252 {
            n838 = Unbundle(w1666) -> (w1667:u8, w1668:u8, w1669:u8, w1670:u8, w1671:u8, w1672:u8, w1673:u8, w1674:u8)  [unwired: 10 out]
            n839 = Build Array(w1667, w1668, w1669, w1670, w1671, w1672, w1673, w1674) -> (w1665:u8[])
            n840 = disable-structure shown="禁用" {
              disable-tunnel: w1682 -> [w1691 _]
              disable-tunnel: [w1690 _] -> w1681
              disable-tunnel: w1680 -> [w1689 _]
              disable-tunnel: w1679 -> [w1688 _]
              disable-tunnel: w1678 -> [w1687 _]
              disable-tunnel: w1677 -> [w1686 _]
              disable-tunnel: w1676 -> [w1685 _]
              disable-tunnel: w1675 -> [w1684 _]
              disable-tunnel: w1665 -> [w1683 _]
              frame Disabled {
                n841 = stacked-sequence {
                  tunnel: w1691 -> [_ w1714]
                  tunnel: [_ w1713] -> w1690
                  tunnel: w1689 -> [w1695 w1712]
                  tunnel: w1688 -> [w1694 w1711]
                  tunnel: w1687 -> [w1693 w1710]
                  tunnel: w1686 -> [_ w1708]
                  tunnel: w1685 -> [_ w1707]
                  tunnel: w1683 -> [_ w1701]
                  tunnel: w1684 -> [w1692 w1696]
                  frame #0 {
                    n842 = dll-call lib="F:/Bluewave New Energy/SVN_Work/AutoTest_TestStand/trunk/AutoTest_TestStand/Driver/ZlgCan/BHN01/AutoBurn/Settings/ControlCAN.dll" fn="VCI_ClearBuffer" label="VCI_Clearbuffer"("DeviceType"=w1695, "DeviceInd"=w1694, "CANInd"=w1693) -> ()  [unwired: 4 in, 5 out]
                    n843 = Flush Queue(queue=w1692) -> ()  [unwired: 1 in, 3 out]
                  }
                  frame #1 {
                    # "FC"
                    n844 = local read "发送的数据"() -> (w1706:i32[])
                    n845 = String Length(string=w1714) -> (length=w1715:i32)
                    n846 = Array Subset(array=w1701, index=1 ("索引"), length=6 ("长度")) -> (w1699:u8[])
                    n847 = Array Size(array=w1708) -> (size(s)=w1709:i32)
                    n848 = Array Subset(array=w1706, index=1 ("索引"), length=6 ("长度")) -> (w1700:i32[])
                    n849 = Greater Than 0?(x=w1715) -> (x > 0?=w1716:bool)
                    n850 = Equal?(x=w1700, y=w1699) -> (x = y?=w1698:bool[])
                    n851 = And Array Elements(Boolean array=w1698) -> (logical AND=w1697:bool)
                    n852 = case shown="假" w1697 {
                      tunnel: w1716 -> [_ w1728]
                      tunnel: w1715 -> [_ w1727]
                      tunnel: w1714 -> [_ w1726]
                      tunnel: [_ w1725] -> w1713
                      tunnel: w1712 -> [_ w1724]
                      tunnel: w1711 -> [_ w1723]
                      tunnel: w1710 -> [_ w1722]
                      tunnel: w1709 -> [_ w1721]
                      tunnel: w1707 -> [_ w1720]
                      tunnel: w1696 -> [_ w1719]
                      frame False {
                        w1717 = "失败" ("布尔文本.文本")
                        w1718 = cluster{u32, u32}[] [{16711680, 0}] ("颜色[4]")
                        n853 = property on="校验" class="Bool (严格)"("Colors [4]"=w1718, "BoolText.Text"=w1717) -> ()  [unwired: 2 in, 2 out]
                        n854 = property on="烧录结果" class="Bool (严格)"("Colors [4]"=w1718, "BoolText.Text"=w1717) -> ()  [unwired: 2 in, 2 out]
                      }
                      frame True {
                        n855 = case shown="假" w1728 {
                          tunnel: w1727 -> [_ w1742]
                          tunnel: w1726 -> [w1729 w1743]
                          tunnel: [w1729 w1741] -> w1725
                          tunnel: w1724 -> [_ w1738]
                          tunnel: w1723 -> [_ w1737]
                          tunnel: w1722 -> [_ w1736]
                          tunnel: w1721 -> [_ _]
                          tunnel: w1720 -> [_ w1732]
                          tunnel: w1719 -> [_ w1730]
                          frame False {
                          }
                          frame True {
                            n856 = Quotient & Remainder(x=w1742, y=12) -> (x-y*floor(x/y)=w1734:i32, floor(x/y)=w1733:i32)
                            n857 = Greater Than 0?(x=w1733) -> (x > 0?=w1744:bool)
                            n858 = case shown="真" w1744 {
                              tunnel: w1743 -> [w1760 w1783]
                              tunnel: w1742 -> [_ w1780]
                              tunnel: ["" w1779] -> w1741
                              tunnel: [w1747 w1778] -> w1739
                              tunnel: w1734 -> [w1757 _]
                              tunnel: [w1748 u8 8 ("DataLen")] -> w1735
                              tunnel: w1732 -> [w1746 _]
                              frame False {
                                n859 = Divide(x=w1757, y=2) -> (x/y=w1752:dbl)
                                "发送数据长度" <- w1752
                                n860 = String Subset(string=w1760, length (rest)=w1757) -> (substring=w1750:string)  [unwired: 1 in]
                                n861 = Increment(x=w1752) -> (x+1=w1756:dbl)
                                n862 = Increment(x=w1756) -> (x+1=w1749:dbl)
                                n863 = Quotient & Remainder(x=w1752, y=2.0) -> (x-y*floor(x/y)=w1754:dbl)  [unwired: 1 out]
                                n864 = Equal?(x=w1754, y=1.0) -> (x = y?=w1751:bool)
                                n865 = case shown="真" w1751 {
                                tunnel: w1750 -> [w1761 w1765]
                                tunnel: w1749 -> [w1762 w1767]
                                tunnel: [w1762 w1766] -> w1748
                                tunnel: [w1761 w1764] -> w1747
                                tunnel: w1746 -> [_ w1763]
                                frame False {
                                }
                                frame True {
                                n866 = case shown="\"主板\"" w1763 {
                                tunnel: w1767 -> [w1771 w1774]
                                tunnel: [w1770 w1774] -> w1766
                                tunnel: w1765 -> [w1769 w1773]
                                tunnel: [w1768 w1773] -> w1764
                                frame "主板" {
                                n867 = Concatenate Strings(w1769, "FF") -> (w1768:string)
                                n868 = Increment(x=w1771) -> (x+1=w1770:dbl)
                                }
                                frame "从板", Default {
                                }
                                }
                                }
                                }
                              }
                              frame True {
                                w1777 = 12 ("长度（剩余）")
                                n869 = Subtract(x=w1780, y=12 ("长度（剩余）")) -> (x-y=w1782:i32)
                                n870 = String Subset(string=w1783, offset (0)=w1777, length (rest)=w1782) -> (substring=w1779:string)
                                n871 = String Subset(string=w1783, length (rest)=w1777) -> (substring=w1778:string)  [unwired: 1 in]
                                n872 = local write "发送数据长度"(6.0 ("发送数据长度")) -> ()
                              }
                            }
                            n873 = call "CAN R&W.vi"("设备类型"=w1738, "设备索引"=w1737, "CAN路数"=w1736, "DataLen"=w1735, "写地址/数据"=enum16{"写地址", "写数据"}."写数据", "Data Input"=w1739, "枚举"=w1732, "queue out"=w1730) -> ("发送的数据"=w1731:i32[])  [unwired: 18 in, 1 out]
                            n874 = local write "发送的数据"(w1731) -> ()
                          }
                        }
                      }
                    }
                  }
                }
              }
              frame Enabled {
              }
            }
          }
          frame 251 {
            n875 = disable-structure shown="禁用" {
              disable-tunnel: w1794 -> [w1823 _]
              disable-tunnel: w1793 -> [w1822 _]
              disable-tunnel: w1792 -> [w1821 _]
              disable-tunnel: [w1819 _] -> w1791
              disable-tunnel: w1790 -> [w1818 _]
              disable-tunnel: [w1816 _] -> w1789
              disable-tunnel: w1788 -> [w1815 _]
              disable-tunnel: w1787 -> [w1814 _]
              disable-tunnel: w1786 -> [w1813 _]
              disable-tunnel: w1785 -> [w1805 _]
              disable-tunnel: w1784 -> [w1796 _]
              frame Disabled {
                w1810 = 1 ("索引")
                # "FB"
                n876 = Unbundle(w1796) -> (w1797:u8, w1798:u8, w1799:u8, w1800:u8, w1801:u8, w1802:u8, w1803:u8, w1804:u8)  [unwired: 10 out]
                n877 = Build Array(w1797, w1798, w1799, w1800, w1801, w1802, w1803, w1804) -> (w1795:u8[])
                n878 = local read "发送数据长度"() -> (w1811:dbl)
                n879 = local read "发送的数据"() -> (w1812:i32[])
                n880 = String Length(string=w1818) -> (length=w1820:i32)
                n881 = Array Subset(array=w1812, index=w1810, length=w1811) -> (w1808:i32[])
                n882 = Array Subset(array=w1795, index=w1810, length=w1810) -> (w1807:u8[])
                n883 = Array Size(array=w1815) -> (size(s)=w1817:i32)
                n884 = Greater Than 0?(x=w1820) -> (x > 0?=w1824:bool)
                n885 = Equal?(x=w1808, y=w1807) -> (x = y?=w1809:bool[])
                n886 = And Array Elements(Boolean array=w1809) -> (logical AND=w1806:bool)
                n887 = case shown="真" w1806 {
                  tunnel: w1824 -> [_ w1840]
                  tunnel: w1823 -> [_ w1839]
                  tunnel: w1822 -> [_ w1838]
                  tunnel: w1821 -> [_ w1837]
                  tunnel: w1820 -> [_ w1836]
                  tunnel: [_ w1835] -> w1819
                  tunnel: w1818 -> [_ w1834]
                  tunnel: w1817 -> [_ w1833]
                  tunnel: [_ w1832] -> w1816
                  tunnel: w1815 -> [_ w1831]
                  tunnel: w1814 -> [_ w1830]
                  tunnel: w1813 -> [_ w1829]
                  tunnel: w1805 -> [_ w1828]
                  tunnel: w1805 -> [_ w1827]
                  frame False {
                    w1825 = "失败" ("布尔文本.文本")
                    w1826 = cluster{u32, u32}[] [{16711680, 0}] ("颜色[4]")
                    n888 = property on="烧录结果" class="Bool (严格)"("Colors [4]"=w1826, "BoolText.Text"=w1825) -> ()  [unwired: 2 in, 2 out]
                    n889 = property on="校验" class="Bool (严格)"("Colors [4]"=w1826, "BoolText.Text"=w1825) -> ()  [unwired: 2 in, 2 out]
                  }
                  frame True {
                    n890 = case shown="真" w1840 {
                      tunnel: w1839 -> [w1853 w1953]
                      tunnel: w1838 -> [w1852 w1952]
                      tunnel: w1837 -> [w1851 w1951]
                      tunnel: w1836 -> [_ w1950]
                      tunnel: w1834 -> [_ w1949]
                      tunnel: [w1850 w1948] -> w1835
                      tunnel: w1834 -> [w1849 _]
                      tunnel: w1833 -> [w1846 _]
                      tunnel: w1831 -> [w1854 _]
                      tunnel: [w1848 w1944] -> w1832
                      tunnel: w1831 -> [w1847 w1944]
                      tunnel: w1830 -> [w1843 w1942]
                      tunnel: w1829 -> [w1842 _]
                      tunnel: w1828 -> [_ w1940]
                      tunnel: w1827 -> [w1841 _]
                      frame False {
                        n891 = Greater?(x=w1846, y=0) -> (0:w1844:bool)
                        n892 = case shown="真" w1844 {
                          tunnel: w1854 -> [_ w1902]
                          tunnel: w1853 -> [w1858 w1905]
                          tunnel: w1852 -> [w1857 w1904]
                          tunnel: w1851 -> [w1861 w1903]
                          tunnel: [w1877 w1901] -> w1850
                          tunnel: w1849 -> [w1877 _]
                          tunnel: [w1876 w1900] -> w1848
                          tunnel: w1847 -> [w1876 _]
                          tunnel: w1843 -> [_ w1893]
                          tunnel: w1842 -> [w1863 _]
                          tunnel: w1841 -> [_ w1891]
                          frame False {
                            w1855 = "成功" ("布尔文本.文本")
                            w1856 = cluster{u32, u32}[] [{6618880, 0}] ("颜色[4]")
                            w1871 = u8 0 ("元素")
                            n893 = flat-sequence {
                              tunnel: w1863 -> [w1888]
                              tunnel: [w1888] -> w1862
                              tunnel: [w1890] -> w1864
                              tunnel: w1862 -> [w1890]
                              frame #0 {
                                n894 = invoke on="开始监控 2" class="Bool" method="Reinit To Default"() -> ()  [unwired: 3 in, 3 out]
                                n895 = local write "TEMP"(FALSE ("TEMP")) -> ()
                              }
                              frame #1 {
                                n896 = Wait (ms)(milliseconds to wait=u32 500 ("等待时间（毫秒）")) -> ()  [unwired: 1 out]
                              }
                            }
                            n897 = Bundle(cluster=w1864, "ID"=u32 0, "TimeStamp"=u8 0 ("RemoteFlag"), "TimeFlag"=u8 1, "SendType"=u8 0 ("DataLen"), "RemoteFlag"=u8 0, "ExternFlag"=u8 0, "DataLen"=u8 1, u8 5 ("元素"), w1871, w1871, w1871) -> (w1875:T1)  [unwired: 7 in]
                            n898 = dll-call lib="F:/Bluewave New Energy/SVN_Work/AutoTest_TestStand/trunk/AutoTest_TestStand/Driver/ZlgCan/BHN01/AutoBurn/Settings/ControlCAN.dll" fn="VCI_Transmit"("DeviceType"=w1858, "DeviceInd"=w1857, "CANInd"=w1861, "pSend"=w1875, "Len"=u32 1) -> (error out=w1860:errorcluster)  [unwired: 5 in, 5 out]
                            n899 = local read "Mode"() -> (w1859:bool)
                            n900 = case shown="假" w1859 {
                              tunnel: w1858 -> [_ w1886]
                              tunnel: w1857 -> [_ w1885]
                              tunnel: w1861 -> [_ w1884]
                              tunnel: w1860 -> [_ w1882]
                              frame False {
                                n901 = flat-sequence {
                                frame #0 {
                                n902 = Wait (ms)(milliseconds to wait=u32 500 ("等待时间（毫秒）")) -> ()  [unwired: 1 out]
                                }
                                frame #1 {
                                n903 = local write "TEMP"(TRUE ("TEMP")) -> ()
                                n904 = local write "连接状态"(TRUE ("CAN连接状态")) -> ()
                                }
                                }
                              }
                              frame True {
                                n905 = invoke on="开始监控" class="Bool" method="Reinit To Default"() -> ()  [unwired: 3 in, 3 out]
                                n906 = local write "连接状态"(FALSE ("CAN连接状态")) -> ()
                                n907 = call "CAN_Init.vi"("设备类型"=w1886, "设备索引"=w1885, "CAN路数"=w1884, "操作类型"=enum16{"初始化CAN", "关闭CAN"}."关闭CAN", 5:w1882) -> ()  [unwired: 14 in, 1 out]
                              }
                            }
                            n908 = property on="烧录结果" class="Bool (严格)"("Colors [4]"=w1856, "BoolText.Text"=w1855) -> ()  [unwired: 2 in, 2 out]
                            n909 = invoke on="Monitor" class="Bool" method="Reinit To Default"() -> ()  [unwired: 3 in, 3 out]
                            n910 = property on="校验" class="Bool (严格)"("Colors [4]"=w1856, "BoolText.Text"=w1855) -> ()  [unwired: 2 in, 2 out]
                          }
                          frame True {
                            w1895 = 100.0 ("y")
                            n911 = Delete From Array(array=w1902, length=1 ("长度"), index=0 ("索引")) -> (array with subset deleted=w1900:string[])  [unwired: 1 out]
                            n912 = local read "大小"() -> (w1898:i32)
                            n913 = Array Size(array=w1900) -> (size(s)=w1899:i32)
                            n914 = Index Array(array=w1902, index=0 ("索引")) -> (element=w1910:string)
                            n915 = Divide(x=w1899, y=w1898) -> (x/y=w1897:dbl)
                            n916 = String Subset(string=w1910, offset (0)=0 ("偏移量(0)"), length (rest)=2 ("长度（剩余）")) -> (substring=w1917:string)
                            n917 = String Subset(string=w1910, offset (0)=2 ("偏移量(0)"), length (rest)=2 ("长度（剩余）")) -> (substring=w1920:string)
                            n918 = Multiply(x=w1897, y=w1895) -> (x*y=w1896:dbl)
                            n919 = Subtract(x=w1895, y=w1896) -> (x-y=w1894:dbl)
                            n920 = Hexadecimal String To Number(string=w1920) -> (number=w1915:u32)  [unwired: 2 in, 1 out]
                            n921 = case shown="\"S1\", 默认" w1917 {
                              tunnel: [4 ("偏移量(0)") 6 ("偏移量(0)")] -> w1909
                              tunnel: w1915 -> [w1932 w1938]
                              tunnel: [w1930 w1936] -> w1914
                              tunnel: [8 ("y") 10 ("y")] -> w1911
                              tunnel: ["S1" "S2"] -> w1906
                              frame "S1", Default {
                                n922 = Subtract(x=w1932, y=3) -> (x-y=w1930:u32)
                              }
                              frame "S2" {
                                n923 = Subtract(x=w1938, y=4) -> (x-y=w1936:u32)
                              }
                            }
                            "地址长度 2" <- w1909
                            n924 = local write "进度"(w1894) -> ()
                            n925 = String Subset(string=w1910, offset (0)=4 ("偏移量(0)"), length (rest)=w1909) -> ()  [unwired: 1 out]
                            n926 = Multiply(x=u32 2, y=w1914) -> (x*y=w1912:u32)
                            "数据长度 2" <- w1912
                            n927 = String Subset(string=w1910, offset (0)=4 ("偏移量(0)"), length (rest)=w1909) -> (substring=w1907:string)
                            n928 = call "CAN R&W.vi"("设备类型"=w1905, "设备索引"=w1904, "CAN路数"=w1903, "DataLen"=u8 8, "写地址/数据"=enum16{"写地址", "写数据"}."写地址", "Data Input"=w1907, "枚举"=w1893, "TYPE"=w1906, "queue out"=w1891) -> ("发送的数据"=w1892:i32[])  [unwired: 17 in, 1 out]
                            n929 = local write "发送的数据"(w1892) -> ()
                            n930 = String Subset(string=w1910, offset (0)=w1911, length (rest)=w1912) -> (substring=w1901:string)
                            "子字符串 2" <- w1901
                          }
                        }
                      }
                      frame True {
                        n931 = Quotient & Remainder(x=w1950, y=12) -> (x-y*floor(x/y)=w1945:i32, floor(x/y)=w1946:i32)
                        n932 = Greater Than 0?(x=w1946) -> (x > 0?=w1955:bool)
                        n933 = case shown="假" w1955 {
                          tunnel: w1949 -> [w1975 w2000]
                          tunnel: w1950 -> [_ w1997]
                          tunnel: ["" w1996] -> w1948
                          tunnel: [w1960 w1995] -> w1943
                          tunnel: w1945 -> [w1973 _]
                          tunnel: [w1961 u8 8 ("DataLen")] -> w1947
                          tunnel: w1944 -> [w1970 _]
                          tunnel: w1942 -> [w1959 _]
                          frame False {
                            n934 = Divide(x=w1973, y=2) -> (x/y=w1958:dbl)
                            n935 = Array Size(array=w1970) -> (size(s)=w1969:i32)
                            n936 = String Subset(string=w1975, length (rest)=w1973) -> (substring=w1963:string)  [unwired: 1 in]
                            n937 = Increment(x=w1958) -> (x+1=w1971:dbl)
                            n938 = Increment(x=w1971) -> (x+1=w1962:dbl)
                            n939 = Equal?(x=0, y=w1969) -> (x = y?=w1957:bool)
                            n940 = Quotient & Remainder(x=w1958, y=2.0) -> (x-y*floor(x/y)=w1966:dbl)  [unwired: 1 out]
                            n941 = local write "发送数据长度"(w1958) -> ()
                            n942 = Equal?(x=w1966, y=1.0) -> (x = y?=w1964:bool)
                            n943 = case shown="真" w1957 {
                              frame False {
                              }
                              frame True {
                                w1976 = "成功" ("布尔文本.文本")
                                w1977 = cluster{u32, u32}[] [{6618880, 0}] ("颜色[4]")
                                n944 = invoke on="Monitor" class="Bool" method="Reinit To Default"() -> ()  [unwired: 3 in, 3 out]
                                n945 = property on="烧录结果" class="Bool (严格)"("Colors [4]"=w1977, "BoolText.Text"=w1976) -> ()  [unwired: 2 in, 2 out]
                                n946 = property on="校验" class="Bool (严格)"("Colors [4]"=w1977, "BoolText.Text"=w1976) -> ()  [unwired: 2 in, 2 out]
                              }
                            }
                            n947 = case shown="假" w1964 {
                              tunnel: w1963 -> [w1978 w1982]
                              tunnel: w1962 -> [w1979 w1984]
                              tunnel: [w1979 w1983] -> w1961
                              tunnel: [w1978 w1981] -> w1960
                              tunnel: w1959 -> [_ w1980]
                              frame False {
                              }
                              frame True {
                                n948 = case shown="\"主板\"" w1980 {
                                tunnel: w1984 -> [w1989 w1991]
                                tunnel: [w1988 w1991] -> w1983
                                tunnel: w1982 -> [w1987 w1990]
                                tunnel: [w1985 w1990] -> w1981
                                frame "主板" {
                                n949 = Concatenate Strings(w1987, "FF") -> (w1985:string)
                                n950 = Increment(x=w1989) -> (x+1=w1988:dbl)
                                }
                                frame "从板", Default {
                                }
                                }
                              }
                            }
                          }
                          frame True {
                            w1994 = 12 ("长度（剩余）")
                            n951 = Subtract(x=w1997, y=12 ("长度（剩余）")) -> (x-y=w1999:i32)
                            n952 = String Subset(string=w2000, offset (0)=w1994, length (rest)=w1999) -> (substring=w1996:string)
                            n953 = String Subset(string=w2000, length (rest)=w1994) -> (substring=w1995:string)  [unwired: 1 in]
                            n954 = local write "发送数据长度"(6.0 ("发送数据长度")) -> ()
                          }
                        }
                        n955 = call "CAN R&W.vi"("设备类型"=w1953, "设备索引"=w1952, "CAN路数"=w1951, "DataLen"=w1947, "写地址/数据"=enum16{"写地址", "写数据"}."写数据", "Data Input"=w1943, "枚举"=w1942, "queue out"=w1940) -> ("发送的数据"=w1941:i32[])  [unwired: 18 in, 1 out]
                        n956 = local write "发送的数据"(w1941) -> ()
                      }
                    }
                  }
                }
              }
              frame Enabled {
              }
            }
          }
          frame 1, Default {
            (unwired) TRUE
            n957 = disable-structure shown="禁用" {
              disable-tunnel: w2003 -> [w2011 _]
              disable-tunnel: w2002 -> [w2007 _]
              disable-tunnel: w2001 -> [w2006 _]
              frame Disabled {
                # "040000"
                n958 = local read "请选择板号"() -> (w2010:u16)
                n959 = Increment(x=w2010) -> (x+1=w2009:u16)
                n960 = Subtract(x=w2011, y=w2009) -> (x-y=w2008:u32)
                n961 = case shown="0, 默认" w2008 {
                  tunnel: w2007 -> [_ w2012 w2017]
                  tunnel: w2006 -> [_ _ w2016]
                  frame 0, Default {
                  }
                  frame 67108864 {
                    n962 = local write "Life"(w2012) -> ()
                  }
                  frame 67174400 {
                    n963 = Join Numbers(hi=w2017, lo=w2016) -> ((hi.lo)=w2015:u16)
                    n964 = Divide(x=w2015, y=u16 10) -> (x/y=→"总电压":dbl)
                  }
                }
              }
              frame Enabled {
              }
            }
          }
        }
        "VCI_CAN_OBJ_R 2" <- w736
      }
    }
    n965 = local read "退出？(T)"() -> (w715:bool)
  }
  n966 = local write "CAN状态"(w7) -> ()
  n967 = local write "连接状态"(w7) -> ()
  n968 = property on="手动进入编程模式" class="Bool (严格)"("DisabledEnum"=T3."Disabled and Grayed Out" ("禁用")) -> ()  [unwired: 2 in, 2 out]
  n969 = local write "开始下载数据"(FALSE ("开始下载数据")) -> ()
  n970 = Release Queue(queue=w9, error in (no error)=w8) -> ()  [unwired: 1 in, 3 out]
  n971 = local write "start"(u32 0 ("start")) -> ()
  n972 = Build Array(cluster{u32, u32} {0, 0}) -> (w32:cluster{u32, u32}[])
  n973 = local write "Info："("" ("字符串")) -> ()
  n974 = local write "进入烧录"(FALSE ("进入烧录")) -> ()
  n975 = property on="MD5校验" class="Bool (严格)"("Colors [4]"=w32, "BoolText.Text"="失败" ("布尔文本.文本")) -> ()  [unwired: 2 in, 2 out]
  n976 = local write "子数组"(string[] ["  "] ("子数组")) -> ()
  n977 = local write "发送数据长度"(0.0 ("发送数据长度")) -> ()
  n978 = local write "擦除完成"(w42) -> ()
  n979 = local write "进入烧录模式"(w42) -> ()
  "连接状态" <- FALSE ("CAN连接状态")
  "CAN数据" <- FALSE ("烧录中")
  "进度" <- u8 0 ("进度")
  "烧录结果" <- FALSE ("烧录完成")
  "Mode" <- TRUE ("Mode")
  "update flag" <- FALSE
  "退出？(T)" <- FALSE ("退出？(T)")
